vi "LIN_Demo.vi"(11 "Receive":string="LIN_Demo") -> ()   [LabVIEW 2014]
uses:
  TSMaster_API/LIN_Function/Typedef/TSLIN_SendHead.ctl
  <vilib>/Utility/miscctls.llb/LVPointTypeDef.ctl
  TSMaster_API/LIN_Function/Typedef/TLibLIN.ctl
  TSMaster_API/LIN_Function/Typedef/TSLIN_Transmit.ctl
  TSMaster_API/All_Control/Typedef/Hardware Type.ctl
  Utilities/Typedef/Hardware_Subtype.ctl
  TSMaster_API/LIN_Function/Typedef/TSLIN_SetData.ctl
  TSMaster_API/LIN_Function/Typedef/TSLIN_LIN_Set.ctl
  TSMaster_API/All_Control/Typedef/Blf_Log.ctl
  TSMaster_API/LIN_Function/Typedef/TSLIN_LIN Schedule_Table.ctl
  TSMaster_API/LIN_Function/Typedef/TSLIN_Config.ctl
  TSMaster_API/LIN_Function/Typedef/TSLIN_Data.ctl
  TSMaster_API/DataBase/Typedef/FlexRay/TFlexRaySignal.ctl
  TSMaster_API/DataBase/Typedef/LIN/TLINSignal.ctl
  TSMaster_API/DataBase/Typedef/CAN/TCANSignal.ctl
  TSMaster_API/DataBase/Typedef/TDBSignalProperties.ctl
  TSMaster_API/DataBase/Typedef/TDBFrameProperties.ctl
  TSMaster_API/DataBase/Typedef/TDBECUProperties.ctl
  TSMaster_API/DataBase/Typedef/TDBProperties.ctl
  <vilib>/regexp/Match Regular Expression.xnode
  TSMaster_API/DataBase/Typedef/DataBase_array.ctl
  TSMaster_API/DataBase/Typedef/DataBase_array_index.ctl
panel:
  out "DataBase_array":T1
  in  "Diagram shown":bool
  in  "Stop Log":bool
  in  "Start Log":bool
  in  "log":i32(listbox)
  in  "Config":bool
  in  "选项卡控件":enum32{"Setting", "Send&Receie", "LDF_Load"}(tab)
  in  "CH_Mapping":bool
  in  "Set Node":bool
  in  "TS_Mapping":bool
  in  "BLF_Log_PATH":path
  in  "DLL_PATH":path
  in  "Channels used":u16(ring)=1 items=["1 Channel"=1, "2 Channels"=2, "3 Channels"=3, "4 Channels"=4, "5 Channels"=5, "6 Channels"=6, "7 Channels"=7, "8 Channels"=8, "9 Channels"=9, "10 Channels"=10, "11 Channels"=11, "12 Channels"=12, "13 Channels"=13, "14 Channels"=14, "15 Channels"=15, "16 Channels"=16]
  in  "LIN_Data.LIN_Set_Array":T9[](array[typedef]) {"Set_node_funtiontype" items=["MasterNode", "SlaveNode", "MonitorNote"]; "Set"."Hardware Type" items=["BUS_UNKNOWN_TYPE", "TS_TCP_DEVICE", "XL_USB_DEVICE", "TS_USB_DEVICE", "PEAK_USB_DEVICE", "KVASER_USB_DEVICE", "ZLG_USB_DEVICE", "ICS_USB_DEVICE", "TS_TC1005_DEVICE", "CANABLE_USB_DEVICE", "TS_WIRELESS_OBD", "TS_USB_DEVICE_EX", "IXXAT_USB_DEVICE", "TS_ETH_IF_DEVICE", "TS_USB_IF_DEVICE", "BUS_DEV_TYPE_COUNT"]; "Set"."AHwChannel" items=["CHN1", "CHN2", "CHN3", "CHN4", "CHN5", "CHN6", "CHN7", "CHN8", "CHN9", "CHN10", "CHN11", "CHN12", "CHN13", "CHN14", "CHN15", "CHN16", "CHN17", "CHN18", "CHN19", "CHN20", "CHN21", "CHN22", "CHN23", "CHN24", "CHN25", "CHN26", "CHN27", "CHN28", "CHN29", "CHN30", "CHN31", "CHN32"]; "Set"."AAppChannel" items=["CHN1", "CHN2", "CHN3", "CHN4", "CHN5", "CHN6", "CHN7", "CHN8", "CHN9", "CHN10", "CHN11", "CHN12", "CHN13", "CHN14", "CHN15", "CHN16", "CHN17", "CHN18", "CHN19", "CHN20", "CHN21", "CHN22", "CHN23", "CHN24", "CHN25", "CHN26", "CHN27", "CHN28", "CHN29", "CHN30", "CHN31", "CHN32"]; "Set"."AProtocol" items=["Lin_Protocol_13", "Lin_Protocol_20", "Lin_Protocol_21", "Lin_Protocol_J2602"]}
  in  "Export":bool
  in  "Import":bool
  in  "Fold Data":bool
  out "BufferCount":i32
  in  "REC_Channel":i32(ring) items=["CHN1", "CHN2", "CHN3", "CHN4", "CHN5", "CHN6", "CHN7", "CHN8", "CHN9", "CHN10", "CHN11", "CHN12", "CHN13", "CHN14", "CHN15", "CHN16", "CHN17", "CHN18", "CHN19", "CHN20", "CHN21", "CHN22", "CHN23", "CHN24", "CHN25", "CHN26", "CHN27", "CHN28", "CHN29", "CHN30", "CHN31", "CHN32"]
  in  "DIS_REC":bool
  in  "Pause":bool
  in  "Rx/TX":enum16{"Rx", "Tx"}(ring)
  in  "ALINId":u32 format="%.0x"
  in  "ALINDLC":u32 format="%.0x"
  in  "Clear":bool
  in  "LIN_Data_0":i32(listbox)=-1
  in  "LIN_DATA":T13 {"Data7" format="%x"; "Data6" format="%x"; "Data5" format="%x"; "Data4" format="%x"; "Data3" format="%x"; "Data2" format="%x"; "Data1" format="%x"; "Data0" format="%x"}
  in  "Read Message Type":T14(ring)=enum."Receive&send messages"
  out "Receive Status":bool
  out "program loop":i32
  in  "Channel":i32(ring) items=["CHN1", "CHN2", "CHN3", "CHN4", "CHN5", "CHN6", "CHN7", "CHN8", "CHN9", "CHN10", "CHN11", "CHN12", "CHN13", "CHN14", "CHN15", "CHN16", "CHN17", "CHN18", "CHN19", "CHN20", "CHN21", "CHN22", "CHN23", "CHN24", "CHN25", "CHN26", "CHN27", "CHN28", "CHN29", "CHN30", "CHN31", "CHN32"]
  in  "Tag":T15(tab)
  in  "LIN_Schedule_Tab":bool
  in  "Cycle":bool=TRUE
  in  "SendHead&Receive":bool
  out "Successful ?":bool
  in  "ATimeoutMs":i32=200
  in  "Send_Frame":bool
  out "successful ？":bool
  in  "Cycle 2":bool=TRUE
  in  "async&sync":enum16{"async", "sync"}(ring)
  in  "Timeout":u16
  out "Laod LDF Successful?":bool caption="Laod BDC Successful?"
  in  "LDF Tab":enum32{"Message", "Signal"}(tab) caption="Tab Control 2"
  in  "Message Table":string[][](table)=[["Name", ""], ["Data Length", ""], ["Identifier", ""], ["", ""], ["", ""], ["", ""], ["", ""]]
  in  "Signal Table":string[][](table)=[["Name", ""], ["Length", ""], ["Endian", ""], ["DataType", ""], ["FStartBit", ""], ["Factor", ""], ["Offset", ""], ["", ""], ["", ""], ["", ""], ["", ""]]
  in  "Unload":bool
  in  "Load_LDF":bool
  in  "LDF loading channel":i32(ring) items=["CHN1", "CHN2", "CHN3", "CHN4", "CHN5", "CHN6", "CHN7", "CHN8", "CHN9", "CHN10", "CHN11", "CHN12", "CHN13", "CHN14", "CHN15", "CHN16", "CHN17", "CHN18", "CHN19", "CHN20", "CHN21", "CHN22", "CHN23", "CHN24", "CHN25", "CHN26", "CHN27", "CHN28", "CHN29", "CHN30", "CHN31", "CHN32"]
  in  "Tree control":string(tree)
  in  "LDF Path":path
  out "Connect ?":bool
  in  "Disconnect":bool
  in  "Connect":bool
  in  "STOP":bool
  # "LIN_Demo"
  # "Please click the 'Config' button first,Don't click \"Connect\""
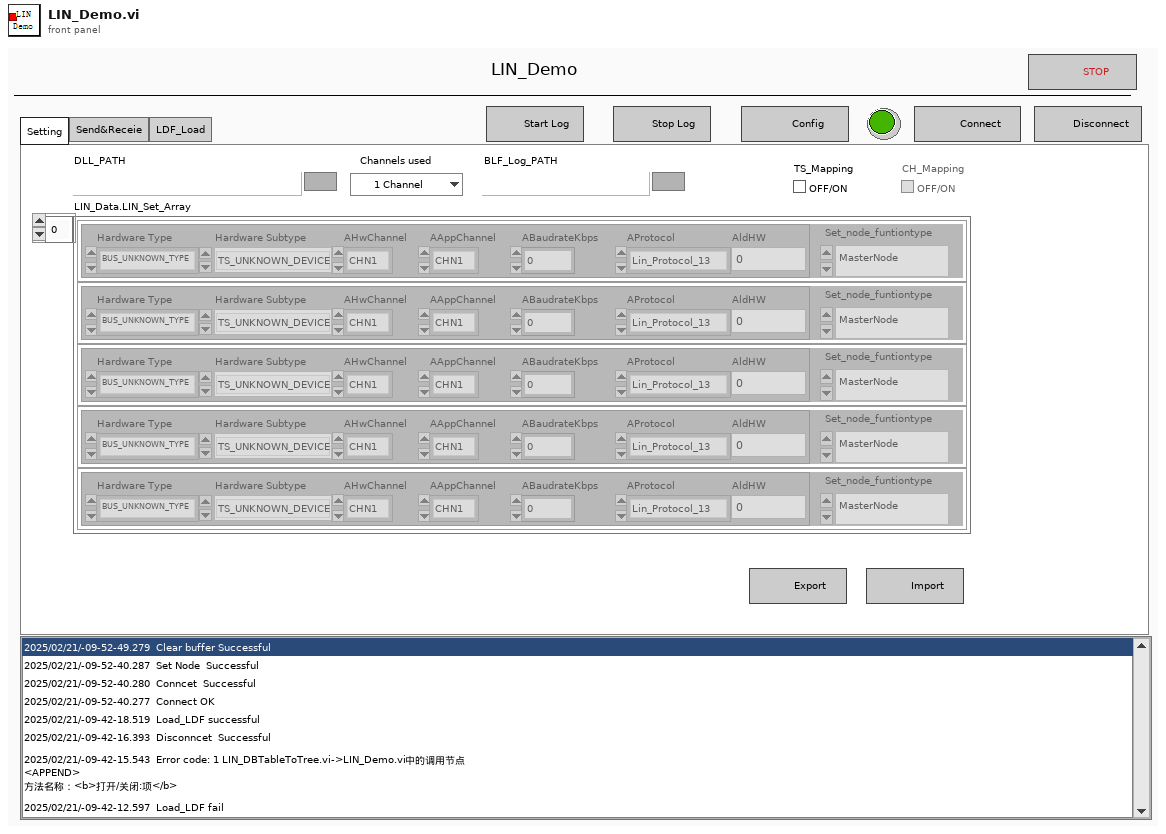
[diagram p1: front panel]
types:
  T1 = typedef "DataBase_array.ctl" = cluster{"db_properties":T2, "ECU_array":cluster{"TDBECUProperties":T3, "TX_Frame_array":cluster{"Frame_Properties":T4, "signal_array":T5[]}[], "RX_Frame_array":cluster{"Frame_Properties":T4, "signal_array":T5[]}[]}[]}[]
  T2 = typedef "TDBProperties.ctl" = cluster{"FDBIndex":i32, "FSignalCount":i32, "FFrameCount":i32, "FECUCount":i32, "FSupportedChannelMask":u64, "FName":cluster{"数值":u64, "数值 2":u64, "数值 3":u64, "数值 4":u64, "数值 5":u64, "数值 6":u64, "数值 7":u64, "数值 8":u64, "数值 9":u64, "数值 10":u64, "数值 11":u64, "数值 12":u64, "数值 13":u64, "数值 14":u64, "数值 15":u64, "数值 16":u64, "数值 17":u64, "数值 18":u64, "数值 19":u64, "数值 20":u64, "数值 21":u64, "数值 22":u64, "数值 23":u64, "数值 24":u64, "数值 25":u64, "数值 26":u64, "数值 27":u64, "数值 28":u64, "数值 29":u64, "数值 30":u64, "数值 31":u64, "数值 32":u64, "数值 33":u64, "数值 34":u64, "数值 35":u64, "数值 36":u64, "数值 37":u64, "数值 38":u64, "数值 39":u64, "数值 40":u64, "数值 41":u64, "数值 42":u64, "数值 43":u64, "数值 44":u64, "数值 45":u64, "数值 46":u64, "数值 47":u64, "数值 48":u64, "数值 49":u64, "数值 50":u64, "数值 51":u64, "数值 52":u64, "数值 53":u64, "数值 54":u64, "数值 55":u64, "数值 56":u64, "数值 57":u64, "数值 58":u64, "数值 59":u64, "数值 60":u64, "数值 61":u64, "数值 62":u64, "数值 63":u64, "数值 64":u64}, "FComment":cluster{"数值":u64, "数值 2":u64, "数值 3":u64, "数值 4":u64, "数值 5":u64, "数值 6":u64, "数值 7":u64, "数值 8":u64, "数值 9":u64, "数值 10":u64, "数值 11":u64, "数值 12":u64, "数值 13":u64, "数值 14":u64, "数值 15":u64, "数值 16":u64, "数值 17":u64, "数值 18":u64, "数值 19":u64, "数值 20":u64, "数值 21":u64, "数值 22":u64, "数值 23":u64, "数值 24":u64, "数值 25":u64, "数值 26":u64, "数值 27":u64, "数值 28":u64, "数值 29":u64, "数值 30":u64, "数值 31":u64, "数值 32":u64, "数值 33":u64, "数值 34":u64, "数值 35":u64, "数值 36":u64, "数值 37":u64, "数值 38":u64, "数值 39":u64, "数值 40":u64, "数值 41":u64, "数值 42":u64, "数值 43":u64, "数值 44":u64, "数值 45":u64, "数值 46":u64, "数值 47":u64, "数值 48":u64, "数值 49":u64, "数值 50":u64, "数值 51":u64, "数值 52":u64, "数值 53":u64, "数值 54":u64, "数值 55":u64, "数值 56":u64, "数值 57":u64, "数值 58":u64, "数值 59":u64, "数值 60":u64, "数值 61":u64, "数值 62":u64, "数值 63":u64, "数值 64":u64}, "FFlags":u32, "FDBId":u32}
  T3 = typedef "TDBECUProperties.ctl" = cluster{"FDBIndex":i32, "FECUIndex":i32, "FTxFrameCount":i32, "FRxFrameCount":i32, "FName":cluster{"数值":u64, "数值 2":u64, "数值 3":u64, "数值 4":u64, "数值 5":u64, "数值 6":u64, "数值 7":u64, "数值 8":u64, "数值 9":u64, "数值 10":u64, "数值 11":u64, "数值 12":u64, "数值 13":u64, "数值 14":u64, "数值 15":u64, "数值 16":u64, "数值 17":u64, "数值 18":u64, "数值 19":u64, "数值 20":u64, "数值 21":u64, "数值 22":u64, "数值 23":u64, "数值 24":u64, "数值 25":u64, "数值 26":u64, "数值 27":u64, "数值 28":u64, "数值 29":u64, "数值 30":u64, "数值 31":u64, "数值 32":u64, "数值 33":u64, "数值 34":u64, "数值 35":u64, "数值 36":u64, "数值 37":u64, "数值 38":u64, "数值 39":u64, "数值 40":u64, "数值 41":u64, "数值 42":u64, "数值 43":u64, "数值 44":u64, "数值 45":u64, "数值 46":u64, "数值 47":u64, "数值 48":u64, "数值 49":u64, "数值 50":u64, "数值 51":u64, "数值 52":u64, "数值 53":u64, "数值 54":u64, "数值 55":u64, "数值 56":u64, "数值 57":u64, "数值 58":u64, "数值 59":u64, "数值 60":u64, "数值 61":u64, "数值 62":u64, "数值 63":u64, "数值 64":u64}, "FComment":cluster{"数值":u64, "数值 2":u64, "数值 3":u64, "数值 4":u64, "数值 5":u64, "数值 6":u64, "数值 7":u64, "数值 8":u64, "数值 9":u64, "数值 10":u64, "数值 11":u64, "数值 12":u64, "数值 13":u64, "数值 14":u64, "数值 15":u64, "数值 16":u64, "数值 17":u64, "数值 18":u64, "数值 19":u64, "数值 20":u64, "数值 21":u64, "数值 22":u64, "数值 23":u64, "数值 24":u64, "数值 25":u64, "数值 26":u64, "数值 27":u64, "数值 28":u64, "数值 29":u64, "数值 30":u64, "数值 31":u64, "数值 32":u64, "数值 33":u64, "数值 34":u64, "数值 35":u64, "数值 36":u64, "数值 37":u64, "数值 38":u64, "数值 39":u64, "数值 40":u64, "数值 41":u64, "数值 42":u64, "数值 43":u64, "数值 44":u64, "数值 45":u64, "数值 46":u64, "数值 47":u64, "数值 48":u64, "数值 49":u64, "数值 50":u64, "数值 51":u64, "数值 52":u64, "数值 53":u64, "数值 54":u64, "数值 55":u64, "数值 56":u64, "数值 57":u64, "数值 58":u64, "数值 59":u64, "数值 60":u64, "数值 61":u64, "数值 62":u64, "数值 63":u64, "数值 64":u64}}
  T4 = typedef "TDBFrameProperties.ctl" = cluster{"FDBIndex":i32, "FECUIndex":i32, "FFrameIndex":i32, "FIsTx":u8, "FReserved1":u8, "FCycleTimeMs":u16, "TSignalType":i32, "FCANIsDataFrame":u8, "FCANIsStdFrame":u8, "FCANIsEdl":u8, "FCANIsBrs":u8, "FCANIdentifier":i32, "FCANDLC":i32, "FCANDataBytes":i32, "FLINIdentifier":i32, "FLINDLC":i32, "FFRChannelMask":u8, "FFRBaseCycle":u8, "FFRCycleRepetition":u8, "FFRIsStartupFrame":u8, "FFRSlotId":u16, "FFRDLC":u16, "FFRCycleMask":u64, "FSignalCount":i32, "FName":cluster{"数值":u64, "数值 2":u64, "数值 3":u64, "数值 4":u64, "数值 5":u64, "数值 6":u64, "数值 7":u64, "数值 8":u64, "数值 9":u64, "数值 10":u64, "数值 11":u64, "数值 12":u64, "数值 13":u64, "数值 14":u64, "数值 15":u64, "数值 16":u64, "数值 17":u64, "数值 18":u64, "数值 19":u64, "数值 20":u64, "数值 21":u64, "数值 22":u64, "数值 23":u64, "数值 24":u64, "数值 25":u64, "数值 26":u64, "数值 27":u64, "数值 28":u64, "数值 29":u64, "数值 30":u64, "数值 31":u64, "数值 32":u64, "数值 33":u64, "数值 34":u64, "数值 35":u64, "数值 36":u64, "数值 37":u64, "数值 38":u64, "数值 39":u64, "数值 40":u64, "数值 41":u64, "数值 42":u64, "数值 43":u64, "数值 44":u64, "数值 45":u64, "数值 46":u64, "数值 47":u64, "数值 48":u64, "数值 49":u64, "数值 50":u64, "数值 51":u64, "数值 52":u64, "数值 53":u64, "数值 54":u64, "数值 55":u64, "数值 56":u64, "数值 57":u64, "数值 58":u64, "数值 59":u64, "数值 60":u64, "数值 61":u64, "数值 62":u64, "数值 63":u64, "数值 64":u64}, "FComment":cluster{"数值":u64, "数值 2":u64, "数值 3":u64, "数值 4":u64, "数值 5":u64, "数值 6":u64, "数值 7":u64, "数值 8":u64, "数值 9":u64, "数值 10":u64, "数值 11":u64, "数值 12":u64, "数值 13":u64, "数值 14":u64, "数值 15":u64, "数值 16":u64, "数值 17":u64, "数值 18":u64, "数值 19":u64, "数值 20":u64, "数值 21":u64, "数值 22":u64, "数值 23":u64, "数值 24":u64, "数值 25":u64, "数值 26":u64, "数值 27":u64, "数值 28":u64, "数值 29":u64, "数值 30":u64, "数值 31":u64, "数值 32":u64, "数值 33":u64, "数值 34":u64, "数值 35":u64, "数值 36":u64, "数值 37":u64, "数值 38":u64, "数值 39":u64, "数值 40":u64, "数值 41":u64, "数值 42":u64, "数值 43":u64, "数值 44":u64, "数值 45":u64, "数值 46":u64, "数值 47":u64, "数值 48":u64, "数值 49":u64, "数值 50":u64, "数值 51":u64, "数值 52":u64, "数值 53":u64, "数值 54":u64, "数值 55":u64, "数值 56":u64, "数值 57":u64, "数值 58":u64, "数值 59":u64, "数值 60":u64, "数值 61":u64, "数值 62":u64, "数值 63":u64, "数值 64":u64}}
  T5 = typedef "TDBSignalProperties.ctl" = cluster{"FDBIndex":i32, "FECUIndex":i32, "FFrameIndex":i32, "FSignalIndex":i32, "FIsTx":u8, "FReserved1":u8, "FReserved2":u8, "FReserved3":u8, "TSignalType":i32, "TCANSignal":T6, "TLINSignal":T7, "TFlexRaySignal":T8, "FParentFrameId":i32, "FInitValue":dbl, "FName":cluster{"数值":u64, "数值 2":u64, "数值 3":u64, "数值 4":u64, "数值 5":u64, "数值 6":u64, "数值 7":u64, "数值 8":u64, "数值 9":u64, "数值 10":u64, "数值 11":u64, "数值 12":u64, "数值 13":u64, "数值 14":u64, "数值 15":u64, "数值 16":u64, "数值 17":u64, "数值 18":u64, "数值 19":u64, "数值 20":u64, "数值 21":u64, "数值 22":u64, "数值 23":u64, "数值 24":u64, "数值 25":u64, "数值 26":u64, "数值 27":u64, "数值 28":u64, "数值 29":u64, "数值 30":u64, "数值 31":u64, "数值 32":u64, "数值 33":u64, "数值 34":u64, "数值 35":u64, "数值 36":u64, "数值 37":u64, "数值 38":u64, "数值 39":u64, "数值 40":u64, "数值 41":u64, "数值 42":u64, "数值 43":u64, "数值 44":u64, "数值 45":u64, "数值 46":u64, "数值 47":u64, "数值 48":u64, "数值 49":u64, "数值 50":u64, "数值 51":u64, "数值 52":u64, "数值 53":u64, "数值 54":u64, "数值 55":u64, "数值 56":u64, "数值 57":u64, "数值 58":u64, "数值 59":u64, "数值 60":u64, "数值 61":u64, "数值 62":u64, "数值 63":u64, "数值 64":u64}, "FComment":cluster{"数值":u64, "数值 2":u64, "数值 3":u64, "数值 4":u64, "数值 5":u64, "数值 6":u64, "数值 7":u64, "数值 8":u64, "数值 9":u64, "数值 10":u64, "数值 11":u64, "数值 12":u64, "数值 13":u64, "数值 14":u64, "数值 15":u64, "数值 16":u64, "数值 17":u64, "数值 18":u64, "数值 19":u64, "数值 20":u64, "数值 21":u64, "数值 22":u64, "数值 23":u64, "数值 24":u64, "数值 25":u64, "数值 26":u64, "数值 27":u64, "数值 28":u64, "数值 29":u64, "数值 30":u64, "数值 31":u64, "数值 32":u64, "数值 33":u64, "数值 34":u64, "数值 35":u64, "数值 36":u64, "数值 37":u64, "数值 38":u64, "数值 39":u64, "数值 40":u64, "数值 41":u64, "数值 42":u64, "数值 43":u64, "数值 44":u64, "数值 45":u64, "数值 46":u64, "数值 47":u64, "数值 48":u64, "数值 49":u64, "数值 50":u64, "数值 51":u64, "数值 52":u64, "数值 53":u64, "数值 54":u64, "数值 55":u64, "数值 56":u64, "数值 57":u64, "数值 58":u64, "数值 59":u64, "数值 60":u64, "数值 61":u64, "数值 62":u64, "数值 63":u64, "数值 64":u64}}
  T6 = typedef "TCANSignal.ctl" = cluster{"FCANSgnType":u8, "FIsIntel":u8, "FStartBit":i32, "FLength":i32, "FFactor":dbl, "FOffset":dbl}
  T7 = typedef "TLINSignal.ctl" = cluster{"FLINSgnType":u8, "FIsIntel":u8, "FStartBit":i32, "FLength":i32, "FFactor":dbl, "FOffset":dbl}
  T8 = typedef "TFlexRaySignal.ctl" = cluster{"FFRSgnType":u8, "FCompuMethod":u8, "FReserved":u8, "FIsIntel":u8, "FStartBit":i32, "FUpdateBit":i32, "FLength":i32, "FFactor":dbl, "FOffset":dbl, "FActualStartBit":i32, "FActualUpdateBit":i32}
  T9 = typedef "TSLIN_LIN_Set.ctl" = cluster{"Set":T10, "Set_node_funtiontype":i32}
  T10 = typedef "TSLIN_SetData.ctl" = cluster{"Hardware Type":T11, "Hardware Subtype":T12, "AHwChannel":i32, "AAppChannel":i32, "ABaudrateKbps":sgl, "AProtocol":i32, "AldHW":i32}
  T11 = typedef "Hardware Type.ctl" = i32
  T12 = typedef "Hardware_Subtype.ctl" = enum16{"TS_UNKNOWN_DEVICE", "TSCAN_PRO", "TSCAN_Lite1", "TC1001", "TL1001", "TC1011", "TM5011", "TC1002", "TC1014", "TSCANFD2517", "TC1026", "TC1016", "TC1012", "TC1013", "TLog1002", "TC1034", "TC1018", "GW2116", "TC2115", "MP1013", "TC1113", "TC1114", "TP1013", "TC1017", "TP1018", "TF10XX", "TL1004_FD_4_LIN_2", "TE1051", "TP1051", "TP1034", "TTS9015", "TP1026", "TTS1026", "TTS1034", "TTS1018", "TL1011", "TTS1015_LiAuto", "TTS1013_LiAuto", "TTS1016Pro", "TC1054Pro", "TC1054", "TLog1038", "TO1013", "TC1034Pro", "TC1018Pro", "TC1038Pro", "TS_DEV_END"}
  T13 = cluster{"Data0":u8, "Data1":u8, "Data2":u8, "Data3":u8, "Data4":u8, "Data5":u8, "Data6":u8, "Data7":u8}
  T14 = enum16{"Only read received messages", "Receive&send messages"}
  T15 = enum32{"Schedule Table", "SendHead", "SendFrame"}
  T16 = typedef "TLibLIN.ctl" = cluster{"Ch":u8, "Code":u8, "Properties":u8, "FDLC":u8, "ID":u8, "Checksum":u8, "FStaus":u8, "FTimeUS":u64, "FDatas":cluster{"value0":u8, "value 1":u8, "value 2":u8, "value 3":u8, "value 4":u8, "value 5":u8, "value 6":u8, "value 7":u8}}
  T17 = enum8{"Enabled", "Disabled", "Disabled and Grayed Out"}
  T18 = typedef "TSLIN_Data.ctl" = cluster{"Communication message":cluster{"Sender":string, "receiver":string, "message":string, "data":variant}, "LIN_Data":T19, "LIN Data array":T16[], "error in":errorcluster, "REC_Channel":i32, "AsynCall?":bool, "DataBase_array":T24}
  T19 = typedef "TSLIN_Config.ctl" = cluster{"DLL_PATH":path, "Channels used":u16, "Funtiontype":i32, "Rx/TX":enum16{"Rx", "Tx"}, "Read message type":enum16{"Only read received messages", "Receive&send messages"}, "async&sync":enum16{"async", "sync"}, "sync_sendTimeout":u16, "LIN_SendHead":T20, "LIN_Set":T10, "LIN_DATA":cluster{"Data0":u8, "Data1":u8, "Data2":u8, "Data3":u8, "Data4":u8, "Data5":u8, "Data6":u8, "Data7":u8}, "LIN_Set_Array":T9[], "LDF":cluster{"LDF Path":path, "LDF loading channel":i32}, "Blf_Log":T21, "LIN Scheduling Table Array":T22[], "REC_Channel":i32}
  T20 = typedef "TSLIN_SendHead.ctl" = cluster{"ALINIdxchn":u8, "ALINId":u32, "ALINDLC":u32}
  T21 = typedef "Blf_Log.ctl" = cluster{"Blf_Log_PATH":path}
  T22 = typedef "TSLIN_LIN Schedule_Table.ctl" = cluster{"LIN_Transmit":T23, "Delay(ms)":i32}
  T23 = typedef "TSLIN_Transmit.ctl" = cluster{"Channel":i32, "Rx/TX":enum16{"Rx", "Tx"}, "Set_node_funtiontype":i32, "DLC":u32, "ID":u32, "FDatas":cluster{"value0":u8, "value 1":u8, "value 2":u8, "value 3":u8, "value 4":u8, "value 5":u8, "value 6":u8, "value 7":u8}}
  T24 = typedef "DataBase_array_index.ctl" = refnum<vi>
  T25 = typedef "LVPointTypeDef.ctl" = cluster{"Horizontal":i16, "Vertical":i16}
  T26 = cluster{"Sender":string, "receiver":string, "message":string, "data":variant, "LIN Data array":T16[]}
  T27 = cluster{"Sender":string, "receiver":string, "message":string, "data":variant}
  T28 = cluster{"Frame_Properties":T4, "signal_array":T5[]}
  T29 = enum32{"invalid app kind", "Development System", "Run Time System", "Student Edition", "Embedded LabVIEW", "Evaluation", "Custom"}
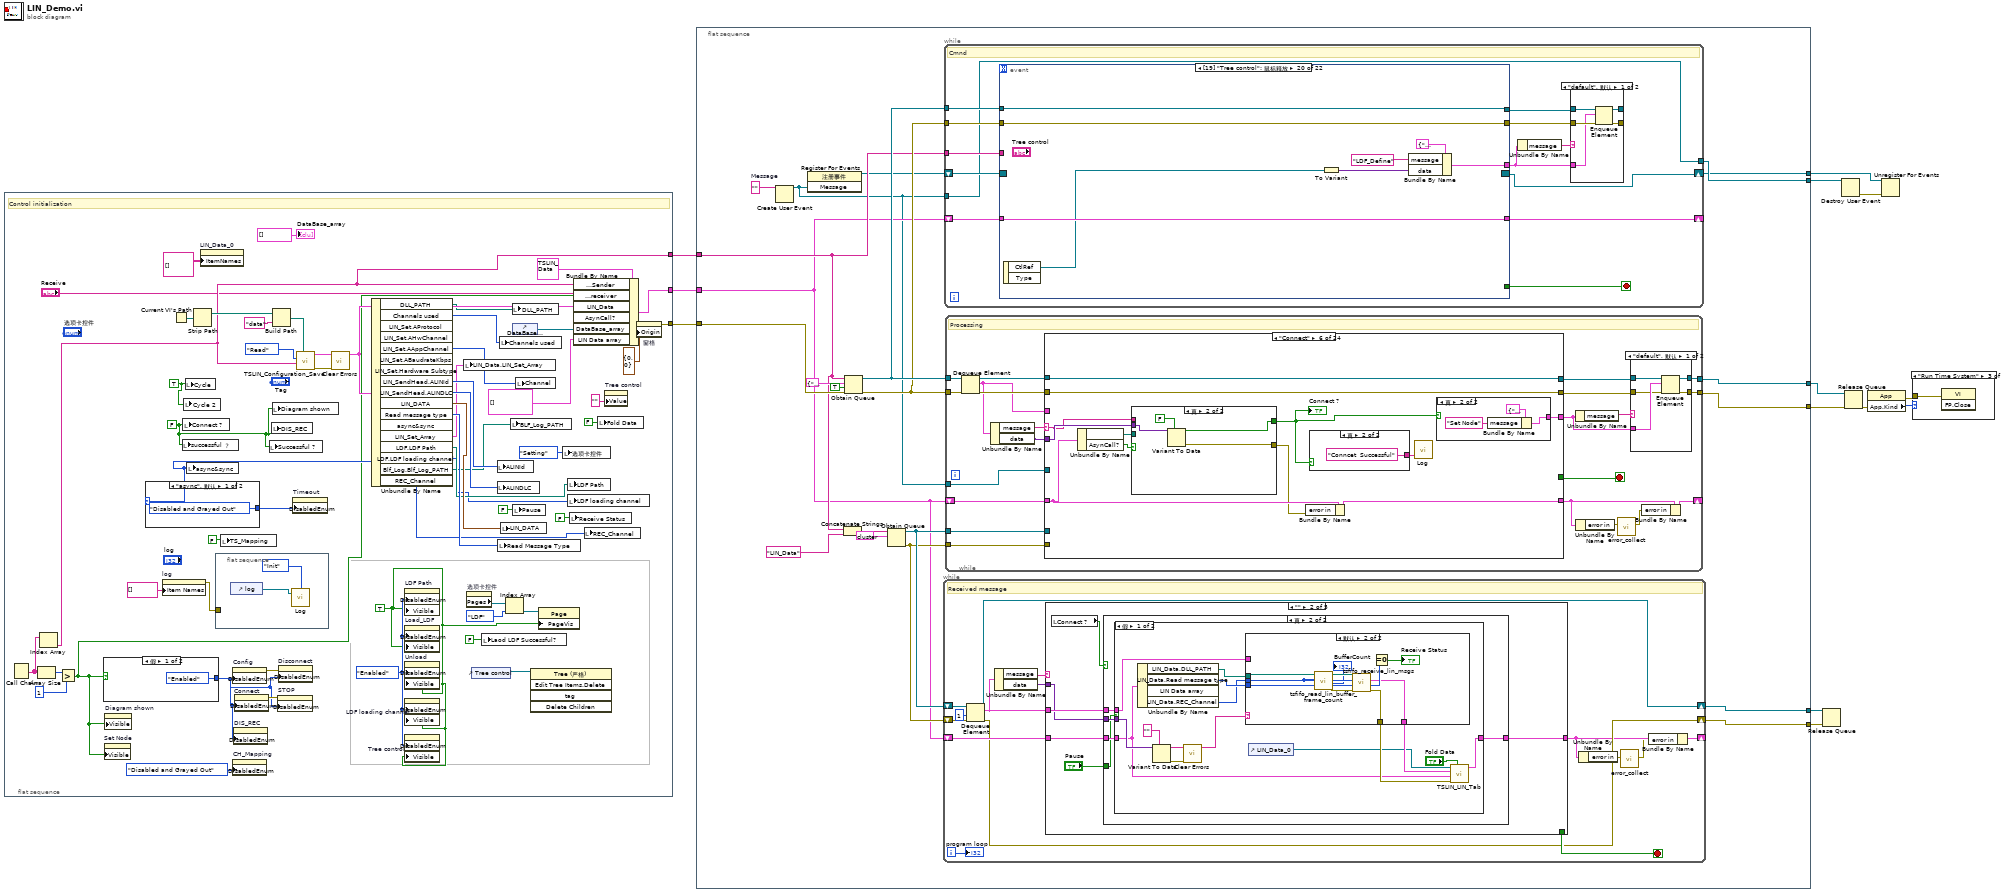
[diagram p0: block diagram]
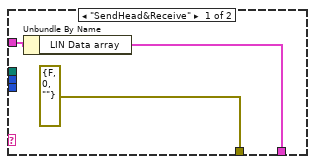
[diagram p4: hidden frame]
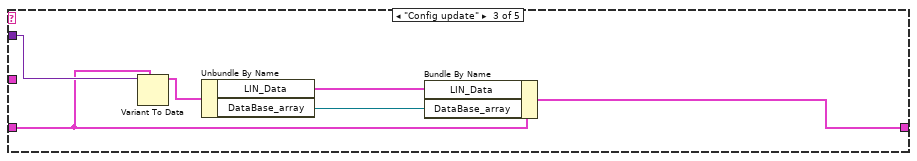
[diagram p6: hidden frame]
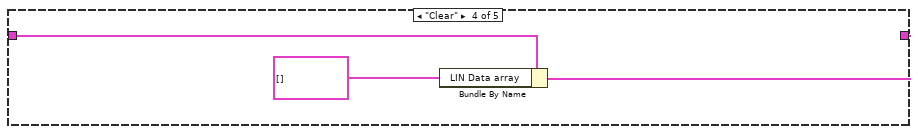
[diagram p7: hidden frame]
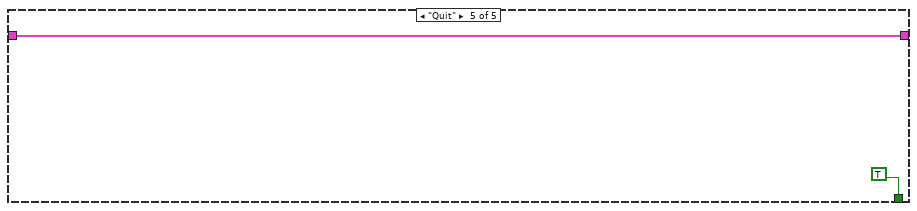
[diagram p8: hidden frame]
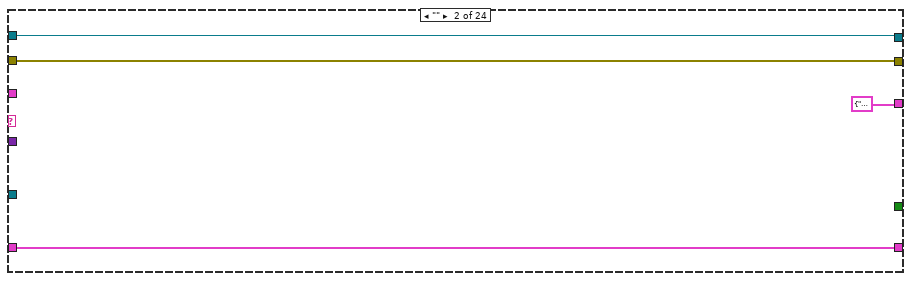
[diagram p11: hidden frame]
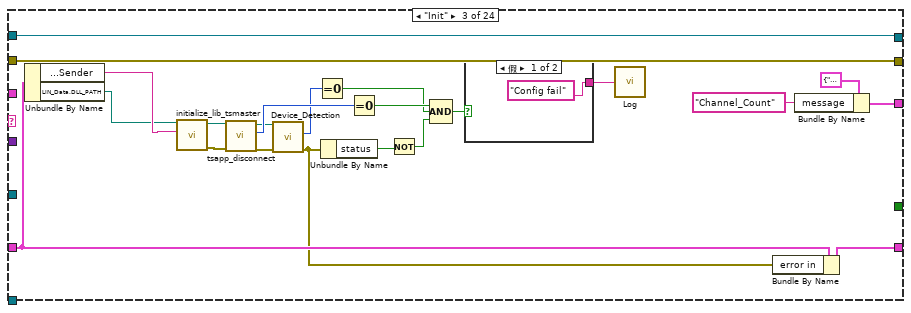
[diagram p12: hidden frame]
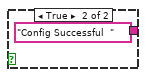
[diagram p13: hidden frame]
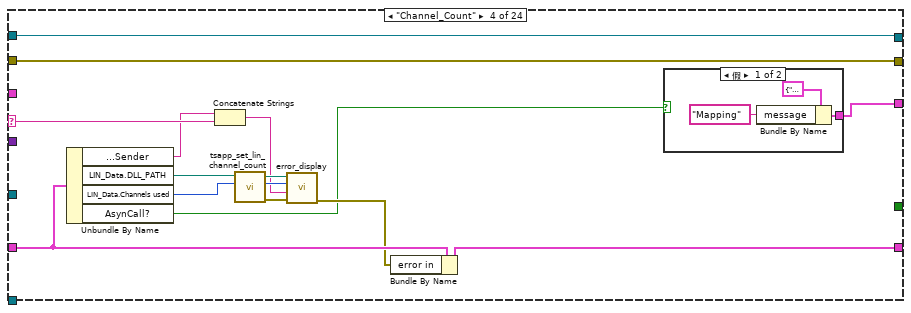
[diagram p14: hidden frame]
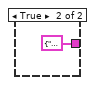
[diagram p15: hidden frame]
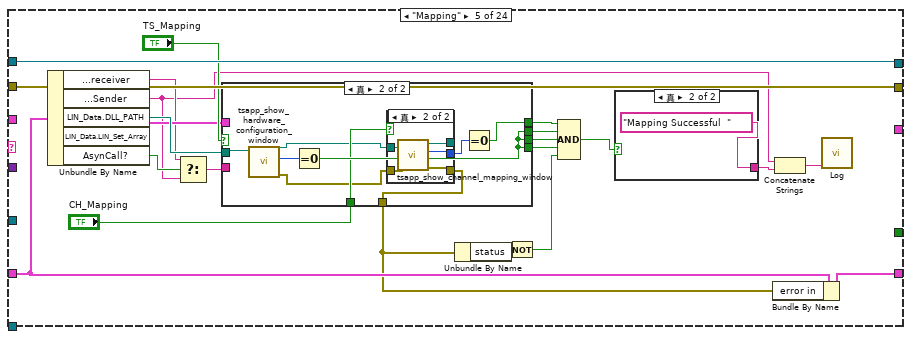
[diagram p16: hidden frame]
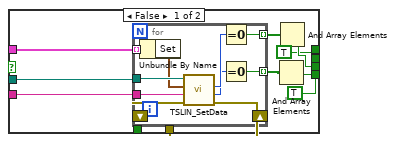
[diagram p17: hidden frame]
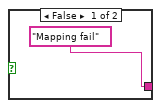
[diagram p19: hidden frame]
diagram:
  n1 = flat-sequence {
    tunnel: [w66] -> w13
    tunnel: [w25] -> w12
    tunnel: [w62] -> w11
    frame #0 {
      w33 = TRUE
      w42 = T17."Enabled" ("禁用")
      w59 = TRUE ("Cycle")
      w27 = FALSE ("Connect ?")
      # "Control initialization"
      n2 = Call Chain() -> (call chain=w26:string[])
      n3 = Array Size(array=w26) -> (size(s)=w29:i32)
      n4 = Index Array(array=w26) -> (element=w25:string)  [unwired: 1 in]
      n5 = Greater?(x=w29, y=1) -> (0:w22:bool)
      n6 = case shown="假" w22 {
        tunnel: [T17."Enabled" ("禁用") T17."Disabled and Grayed Out" ("禁用")] -> w23
        frame False {
        }
        frame True {
        }
      }
      n7 = property on="Set Node" class="Bool"("Visible"=w22) -> ()  [unwired: 2 in, 2 out]
      n8 = property on="Diagram shown" class="Bool (严格)"("Visible"=w22) -> ()  [unwired: 2 in, 2 out]
      n9 = property on="log" class="LstBox (严格)"("Item Names"=string[] [] ("项名")) -> (error out=w40:errorcluster)  [unwired: 2 in, 1 out]
      n10 = Current VI's Path() -> (path=w55:path)
      n11 = local write "successful ？"(w27) -> ()
      n12 = local write "Connect ?"(w27) -> ()
      n13 = local write "Cycle 2"(w59) -> ()
      n14 = local write "Cycle"(w59) -> ()
      n15 = Strip Path(path=w55) -> (stripped path=w53:path)  [unwired: 1 out]
      n16 = property on="LIN_Data_0" class="MCListbox (严格)"("ItemNames"=string[][] [] ("项名")) -> ()  [unwired: 2 in, 2 out]
      n17 = flat-sequence {
        tunnel: w40 -> [_]
        frame #0 {
          n18 = control-ref of="log"() -> (w73:refnum<vi>)
          n19 = call "Log.vi"("Method"=enum16{"Init", "Log"}."Init", "ListBox in"=w73) -> ()  [unwired: 2 in]
        }
      }
      n20 = local write "TS_Mapping"(FALSE ("TS_Mapping")) -> ()
      n21 = property on="Config" class="Bool"("DisabledEnum"=w23) -> (error out=w31:errorcluster)  [unwired: 2 in, 1 out]
      n22 = property on="CH_Mapping" class="Bool (严格)"("DisabledEnum"=T17."Disabled and Grayed Out" ("禁用")) -> ()  [unwired: 2 in, 2 out]
      n23 = property on="DIS_REC" class="Bool (严格)"("DisabledEnum"=w23) -> ()  [unwired: 2 in, 2 out]
      n24 = property on="Connect" class="Bool"("DisabledEnum"=w23) -> (error out=w30:errorcluster)  [unwired: 2 in, 1 out]
      n25 = local write "Successful ?"(w27) -> ()
      n26 = local write "DIS_REC"(w27) -> ()
      n27 = local write "Diagram shown"(w27) -> ()
      n28 = Build Path(base path=w53, name or relative path="data") -> (appended path=w52:path)
      n29 = property on="STOP" class="Bool"(error in=w30, "DisabledEnum"=w23) -> ()  [unwired: 1 in, 2 out]
      n30 = property on="Disconnect" class="Bool"(error in=w31, "DisabledEnum"=w23) -> ()  [unwired: 1 in, 2 out]
      n31 = call "TSLIN_Configuration_Save.vi"("path"=w52, "Config Name"=w25, "Read/Write"=enum16{"Read", "Write"}."Read") -> ("error in (no error) 2"=w48:errorcluster, "LIN_Data out"=w67:T19)  [unwired: 6 in, 1 out]
      n32 = call <vilib>:"Clear Errors.vi"("error in (no error)"=w48) -> ()  [unwired: 5 in, 2 out]
      n33 = Unbundle By Name(w67) -> ("DLL_PATH"=w49:path, "Channels used"=w50:u16, "LIN_Set.AAppChannel"=w68:i32, "LIN_SendHead.ALINId"=w64:u32, "LIN_SendHead.ALINDLC"=w63:u32, "LIN_DATA"=w61:T13, "Read message type"=w57:T14, "async&sync"=w56:enum16{"async", "sync"}, "LIN_Set_Array"=w47:T9[], "LDF.LDF Path"=w45:path, "LDF.LDF loading channel"=w44:i32, "Blf_Log.Blf_Log_PATH"=w36:path, "REC_Channel"=w32:i32)  [unwired: 4 out]
      n34 = case shown="\"async\", 默认" w56 {
        tunnel: [T17."Disabled and Grayed Out" ("禁用") T17."Enabled" ("禁用")] -> w58
        frame "async", Default {
        }
        frame "sync" {
        }
      }
      n35 = local write "async&sync"(w56) -> ()
      n36 = property on="Timeout" class="DigNum (严格)"("DisabledEnum"=w58) -> ()  [unwired: 2 in, 2 out]
      n37 = property on="LDF Path" class="Path"("DisabledEnum"=w42, "Visible"=w33) -> ()  [unwired: 2 in, 2 out]
      n38 = property on="Load_LDF" class="Bool"("DisabledEnum"=w42, "Visible"=w33) -> ()  [unwired: 2 in, 2 out]
      n39 = property on="Unload" class="Bool"("DisabledEnum"=w42, "Visible"=w33) -> ()  [unwired: 2 in, 2 out]
      n40 = property on="LDF loading channel" class="Ring (严格)"("DisabledEnum"=w42, "Visible"=w33) -> ()  [unwired: 2 in, 2 out]
      n41 = property on="Tree control" class="Tree (严格)"("DisabledEnum"=w42, "Visible"=w33) -> ()  [unwired: 2 in, 2 out]
      n42 = local write "LIN_Data.LIN_Set_Array"(w47) -> ()
      n43 = property on="选项卡控件" class="TabCtl (严格)"() -> ("Pages"=w39:refnum<vi>[])  [unwired: 2 in, 2 out]
      n44 = control-ref of="Tree control"() -> (w15:refnum<vi>)
      n45 = local write "Laod LDF Successful?"(FALSE ("Laod LDF Successful?")) -> ()
      n46 = local write "ALINId"(w64) -> ()
      n47 = local write "ALINDLC"(w63) -> ()
      n48 = local write "Read Message Type"(w57) -> ()
      n49 = local write "Channels used"(w50) -> ()
      n50 = local write "LIN_DATA"(w61) -> ()
      n51 = Index Array(array=w39, index=enum32{"Setting", "Send&Receie", "LDF"}."LDF" ("选项卡控件")) -> (element=w37:refnum<vi>)
      n52 = local write "BLF_Log_PATH"(w36) -> ()
      n53 = local write "DLL_PATH"(w49) -> ()
      n54 = control-ref of="DataBase_array"() -> (w16:refnum<vi>)
      n55 = local write "Pause"(FALSE ("Pause")) -> ()
      n56 = local write "Channel"(w68) -> ()
      n57 = invoke class="Tree (严格)" method="Edit Tree Items.Delete"(reference=w15) -> ()  [unwired: 4 in, 5 out]
      n58 = property class="Page"(reference=w37, "PageVis"=w33) -> ()  [unwired: 1 in, 2 out]
      n59 = local write "选项卡控件"(enum32{"Setting", "Send&Receie", "LDF_Load"}."Setting" ("选项卡控件")) -> ()
      n60 = local write "LDF Path"(w45) -> ()
      n61 = local write "LDF loading channel"(w44) -> ()
      n62 = local write "Receive Status"(FALSE ("Receive Status")) -> ()
      n63 = Bundle By Name(cluster=T18 {"Communication message"={"Sender"="", "receiver"="", "message"="", "data"=variant}, "LIN_Data"={"DLL_PATH"=path "", "Channels used"=0, "Funtiontype"=0, "Rx/TX"=enum."Rx", "Read message type"=enum."Only read received messages", "async&sync"=enum."async", "sync_sendTimeout"=0, "LIN_SendHead"={"ALINIdxchn"=0, "ALINId"=0, "ALINDLC"=0}, "LIN_Set"={"Hardware Type"=0, "Hardware Subtype"=enum."TS_UNKNOWN_DEVICE", "AHwChannel"=0, "AAppChannel"=0, "ABaudrateKbps"=0.0, "AProtocol"=0, "AldHW"=0}, "LIN_DATA"={"Data0"=0, "Data1"=0, "Data2"=0, "Data3"=0, "Data4"=0, "Data5"=0, "Data6"=0, "Data7"=0}, "LIN_Set_Array"=[], "LDF"={"LDF Path"=path "", "LDF loading channel"=0}, "Blf_Log"={"Blf_Log_PATH"=path ""}, "LIN Scheduling Table Array"=[], "REC_Channel"=0}, "LIN Data array"=[], "error in"={"status"=FALSE, "code"=0, "source"=""}, "REC_Channel"=0, "AsynCall?"=FALSE, "DataBase_array"=refnum} ("Data"), "Communication message.Sender"=w25, "Communication message.receiver"="Receive", "LIN_Data"=w67, "AsynCall?"=w22, "DataBase_array"=w16, "LIN Data array"=T16[] []) -> (w62:T18)
      n64 = local write "REC_Channel"(w32) -> ()
      n65 = local write "Fold Data"(FALSE ("Fold Data")) -> ()
      n66 = property on="Tree control" class="Tree (严格)"("Value"="" ("Tree control")) -> ()  [unwired: 2 in, 2 out]
      n67 = property on="窗格" class="Pane"("Origin"=T25 {"Horizontal"=0, "Vertical"=0} ("原点")) -> (error out=w66:errorcluster)  [unwired: 2 in, 1 out]
      "DataBase_array" <- T1 [] ("DataBase_array")
    }
  }
  n68 = flat-sequence {
    tunnel: w13 -> [w95]
    tunnel: w12 -> [w89]
    tunnel: w11 -> [w84]
    tunnel: [w81] -> w9
    tunnel: [w80] -> w8
    tunnel: [w79] -> w5
    tunnel: [w78] -> w4
    tunnel: [w77] -> w2
    tunnel: [w76] -> w1
    frame #0 {
      w96 = ""  # Message
      n69 = Create User Event(user event datatype=w96) -> (user event=w82:refnum<user-event>)  [unwired: 1 in, 1 out]
      n70 = register-events(w82) -> (reference out=w83:refnum<event-registration>)  [unwired: 2 in, 1 out]
      n71 = Concatenate Strings(w89, "LIN_Data" ("字符串")) -> (w88:string)
      n72 = Obtain Queue(name (unnamed)=w89, element data type=T27 {"Sender"="", "receiver"="", "message"="", "data"=variant} ("Communication message"), create if not found? (T)=TRUE ("如未找到则创建？(T)"), error in (no error)=w95) -> (queue out=w94:refnum<queue>, error out=w93:errorcluster)  [unwired: 1 in, 1 out]
      n73 = Obtain Queue(name (unnamed)=w88, element data type=T26 {"Sender"="", "receiver"="", "message"="", "data"=variant, "LIN Data array"=[]} ("Communication message")) -> (queue out=w86:refnum<queue>, error out=w85:errorcluster)  [unwired: 3 in, 1 out]
      n74 = while {
        shift-right: [w103] -> w79
        shift-left: w86 -> [w111]
        shift-right: [w102] -> w78
        shift-left: w85 -> [w109]
        shift-right: [w98] -> _
        shift-left: w84 -> [w105]
        i -> [w101]
        stop <- w106 stop-if-true
        # "Received message"
        n75 = Dequeue Element(queue=w111, timeout in ms (-1)=1 ("超时毫秒(-1)"), error in (no error)=w109) -> (queue out=w103:refnum<queue>, element=w104:T26, error out=w102:errorcluster)  [unwired: 1 out]
        n76 = Unbundle By Name(w104) -> ("message"=w108:string, "data"=w107:variant)
        n77 = case shown="\"\"" w108 {
          tunnel: w107 -> [_ w114 w158 _ _]
          tunnel: [_ _ _ _ TRUE] -> w106
          tunnel: w105 -> [w112 w117 w157 w160 w162]
          tunnel: [w112 w116 w156 w159 w162] -> w99
          tunnel: w104 -> [_ w115 _ _ _]
          frame "假", Default {
          }
          frame "" {
            n78 = local read "Connect ?"() -> (w118:bool)
            n79 = case shown="真" w118 {
              tunnel: w117 -> [w119 w121]
              tunnel: [w119 w124] -> w116
              tunnel: w115 -> [_ w123]
              tunnel: w114 -> [_ w122]
              tunnel: "Pause" -> [_ w120]
              frame False {
              }
              frame True {
                n80 = case shown="假" w120 {
                  tunnel: [w136 w152] -> w124
                  tunnel: w123 -> [w135 _]
                  tunnel: w122 -> [w134 _]
                  tunnel: w121 -> [w128 w152]
                  frame False {
                    n81 = Unbundle By Name(w128) -> ("LIN_Data.DLL_PATH"=w138:path, "LIN_Data.Read message type"=w137:T14, "LIN_Data.REC_Channel"=w126:i32)  [unwired: 1 out]
                    n82 = Variant To Data(type="", Variant=w134) -> (data=w132:string, error out=w131:errorcluster)  [unwired: 1 in]
                    n83 = call <vilib>:"Clear Errors.vi"("error in (no error)"=w131) -> ()  [unwired: 5 in, 2 out]
                    n84 = case shown="默认" w132 {
                      tunnel: w138 -> [_ w146]
                      tunnel: w126 -> [_ w144]
                      tunnel: w137 -> [_ w151]
                      tunnel: [w140 w147] -> w130
                      tunnel: w135 -> [w141 _]
                      tunnel: [errorcluster {"status"=FALSE, "code"=0, "source"=""} ("error out") w149] -> w129
                      frame "SendHead&Receive" {
                        n85 = Unbundle By Name(w141) -> ("LIN Data array"=w140:T16[])
                      }
                      frame Default {
                        n86 = call "tsfifo_read_lin_buffer_frame_count.vi"("AAppChannel"=w144, "路径输入"=w146) -> ("错误输出"=w143:errorcluster, "ACount"=→"BufferCount":i32, "路径输出"=w145:path)  [unwired: 6 in, 1 out]
                        n87 = call "tsfifo_receive_lin_msgs.vi"("错误输入（无错误）"=w143, "Read message type"=w151, "AIdxChn"=w144, "路径输入"=w145) -> ("错误输出"=w149:errorcluster, "return"=w150:i32, "ALINBuffer"=w147:T16[])  [unwired: 4 in, 1 out]
                        n88 = Equal To 0?(x=w150) -> (x = 0?=→"Receive Status":bool)
                      }
                    }
                    n89 = control-ref of="LIN_Data_0"() -> (w127:refnum<vi>)
                    n90 = call "TSLIN_LIN_Tab.vi"("Fold Data"="Fold Data", "error in (no error)"=w129, "Data in"=w128, "ALINBuffer"=w130, "MulticolumnListbox in"=w127) -> ("Data out"=w136:T18)  [unwired: 6 in]
                  }
                  frame True {
                  }
                }
              }
            }
          }
          frame "Config update" {
            n91 = Variant To Data(type=w157, Variant=w158) -> (data=w155:T18)  [unwired: 1 in, 1 out]
            n92 = Unbundle By Name(w155) -> ("LIN_Data"=w154:T19, "DataBase_array"=w153:T24)
            n93 = Bundle By Name(cluster=w157, "LIN_Data"=w154, "DataBase_array"=w153) -> (w156:T18)
          }
          frame "Clear" {
            n94 = Bundle By Name(cluster=w160, "LIN Data array"=T16[] []) -> (w159:T18)
          }
          frame "Quit" {
          }
        }
        n95 = Unbundle By Name(w99) -> ("error in"=w100:errorcluster)
        n96 = call "error_collect.vi"("error in (no error)"=w100) -> ("error IO"=w97:errorcluster)  [unwired: 10 in]
        n97 = Bundle By Name(cluster=w99, "error in"=w97) -> (w98:T18)
        "program loop" <- w101
      }
      n98 = while {
        tunnel: w94 -> [w1045]
        tunnel: w93 -> [w1043]
        tunnel: w89 -> [w1039]
        shift-right: [w1036] -> _
        shift-left: w84 -> [w1037]
        shift-right: [w1035] -> w76
        shift-left: w83 -> [w1038]
        tunnel: w82 -> [w1034]
        tunnel: [w1034] -> w77
        stop <- w1046 stop-if-true
        # "Cmnd"
        n99 = event shown="[19] \"Tree control\": 鼠标释放" {
          selector: w1038 -> [_ _ _ _ _ _ _ _ _ _ _ _ _ _ _ _ _ _ _ _ _ _]
          dyn-events: [_ _ _ _ _ _ _ _ _ _ _ _ _ _ _ _ _ _ _ _ _ _] -> w1035
          timeout: _ -> [_ _ _ _ _ _ _ _ _ _ _ _ _ _ _ _ _ _ _ _ _ _]
          tunnel: [_ _ _ _ _ _ _ _ _ _ _ _ _ _ _ _ _ _ w1196 _ w1214 TRUE ("放弃？")] -> w1046
          tunnel: w1045 -> [w1056 w1063 w1069 w1074 w1080 w1084 w1092 w1104 w1113 w1121 w1125 w1151 w1161 w1167 w1173 w1179 w1185 w1192 w1199 w1207 w1213 w1218]
          tunnel: [w1056 w1063 w1069 w1074 w1080 w1084 w1092 w1104 w1113 w1121 w1125 w1151 w1161 w1167 w1173 w1179 w1185 w1192 w1199 w1207 w1213 w1218] -> w1044
          tunnel: [_ w1061 w1064 _ T27 {"Sender"="", "receiver"="", "message"="Connect", "data"=variant} ("Communication message") T27 {"Sender"="", "receiver"="", "message"="Disconnect", "data"=variant} ("Communication message") w1086 w1100 w1108 w1116 T27 {"Sender"="", "receiver"="", "message"="Clear", "data"=variant} ("Communication message") w1144 w1156 w1163 w1168 w1174 w1180 w1187 T27 {"Sender"="", "receiver"="", "message"="eee", "data"=variant} ("Communication message") w1201 w1209 T27 {"Sender"="", "receiver"="", "message"="Quit", "data"=variant} ("Communication message")] -> w1041
          tunnel: [w1055 w1057 w1068 w1073 w1079 w1083 w1091 w1103 w1112 w1120 w1124 w1140 w1160 w1166 w1172 w1178 w1184 w1191 w1194 w1206 w1211 w1216] -> w1042
          tunnel: w1043 -> [w1055 w1057 w1068 w1073 w1079 w1083 w1091 w1103 w1112 w1120 w1124 w1140 w1160 w1166 w1172 w1178 w1184 w1191 w1194 w1206 w1211 w1216]
          tunnel: w1039 -> [_ _ _ _ _ _ _ _ _ _ _ _ _ _ _ _ _ _ _ _ _ _]
          tunnel: w1037 -> [w1054 w1058 w1067 w1072 w1078 w1082 w1090 w1102 w1111 w1119 w1123 w1150 w1159 w1165 w1171 w1177 w1183 w1190 w1195 w1205 w1212 w1217]
          tunnel: [w1054 w1058 w1067 w1072 w1078 w1082 w1090 w1102 w1111 w1119 w1123 w1143 w1159 w1165 w1171 w1177 w1183 w1190 w1195 w1205 w1212 w1217] -> w1036
          event Timeout {
            n100 = event-data() -> ()  [unwired: 1 in, 3 out]
          }
          event "Config": Value Change {
            n101 = event-data() -> ()  [unwired: 1 in, 1 out]
            n102 = To Variant(anything=w1058) -> (Variant=w1059:variant)
            n103 = Bundle By Name(cluster=T27 {"Sender"="", "receiver"="", "message"="", "data"=variant} ("Communication message"), "message"="Init", "data"=w1059) -> (w1061:T27)
          }
          event "Set Node": Value Change {
            n104 = event-data() -> ()  [unwired: 1 in, 1 out]
            n105 = Bundle By Name(cluster=T27 {"Sender"="", "receiver"="", "message"="", "data"=variant} ("Communication message"), "message"="Set Node") -> (w1064:T27)
          }
          event "TS_Mapping": Value Change {
            n106 = event-data() -> ("NewVal"=w1070:bool)  [unwired: 1 in]
            n107 = case shown="假" w1070 {
              tunnel: [T17."Disabled and Grayed Out" ("禁用") T17."Enabled" ("禁用")] -> w1071
              frame False {
              }
              frame True {
              }
            }
            n108 = property on="CH_Mapping" class="Bool (严格)"("DisabledEnum"=w1071) -> ()  [unwired: 2 in, 2 out]
          }
          event "Connect": Value Change {
            n109 = event-data() -> ()  [unwired: 1 in, 1 out]
          }
          event "Disconnect": Value Change {
            n110 = event-data() -> ()  [unwired: 1 in, 1 out]
          }
          event "DIS_REC": Value Change {
            n111 = event-data() -> ("NewVal"=w1085:bool)  [unwired: 1 in, 5 out]
            n112 = To Variant(anything=w1085) -> (Variant=w1087:variant)
            n113 = Bundle By Name(cluster=T27 {"Sender"="", "receiver"="", "message"="", "data"=variant} ("Communication message"), "message"="DIS_REC", "data"=w1087) -> (w1086:T27)
          }
          event "SendHead&Receive": Value Change {
            n114 = event-data() -> ()  [unwired: 1 in, 1 out]
            n115 = property on="Rx/TX" class="Enum (严格)"("Val(Sgnl)"=enum16{"Rx", "Tx"}."Rx" ("值(信号)")) -> ()  [unwired: 2 in, 2 out]
            n116 = Select(t=T17."Disabled and Grayed Out" ("禁用"), s="Cycle", f=T17."Enabled" ("禁用")) -> (s? t:f=w1096:T17)
            n117 = To Variant(anything="Cycle") -> (Variant=w1098:variant)
            n118 = property on="REC_Channel" class="Ring (严格)"("DisabledEnum"=w1096) -> ()  [unwired: 2 in, 2 out]
            n119 = Bundle By Name(cluster=T27 {"Sender"="", "receiver"="", "message"="SendHead&Receive", "data"=variant} ("Communication message"), "message"="SendHead&Receive", "data"=w1098) -> (w1100:T27)
          }
          event "Send_Frame": Value Change {
            # "点击后，若发送成功显示闪烁\nAfter clicking, if the sending is successful, it will flash"
            n120 = event-data() -> ()  [unwired: 1 in, 1 out]
            n121 = property on="Rx/TX" class="Enum (严格)"("Val(Sgnl)"=enum16{"Rx", "Tx"}."Tx" ("值(信号)")) -> ()  [unwired: 2 in, 2 out]
            n122 = flat-sequence {
              frame #0 {
                n123 = local write "successful ？"(FALSE ("successful ？")) -> ()
              }
              frame #1 {
                n124 = Wait (ms)(milliseconds to wait=u32 50 ("等待时间（毫秒）")) -> ()  [unwired: 1 out]
              }
            }
            n125 = To Variant(anything="Cycle 2") -> (Variant=w1107:variant)
            n126 = Bundle By Name(cluster=T27 {"Sender"="", "receiver"="", "message"="SendHead&Receive", "data"=variant} ("Communication message"), "message"="Send_Frame", "data"=w1107) -> (w1108:T27)
          }
          event "LIN_Schedule_Tab": Value Change {
            n127 = event-data() -> ()  [unwired: 1 in, 1 out]
            n128 = Bundle By Name(cluster=T27 {"Sender"="", "receiver"="", "message"="SendHead&Receive", "data"=variant} ("Communication message"), "message"="LIN_Schedule_Tab") -> (w1116:T27)
          }
          event "Clear": Value Change {
            n129 = event-data() -> ()  [unwired: 1 in, 1 out]
          }
          event "DLL_PATH", "Channel", "ALINId", "ALINDLC", "Rx/TX", "LIN_DATA", "Timeout", "async&sync", "Read Message Type", "LIN_Data.LIN_Set_Array", "LDF Path", "LDF loading channel", "BLF_Log_PATH", "Channels used", "REC_Channel": Value Change {
            # "Update data when control value changes"
            n130 = event-data() -> ()  [unwired: 1 in, 1 out]
            n131 = Bundle By Name(cluster=T20 {"ALINIdxchn"=0, "ALINId"=0, "ALINDLC"=0} ("LIN_Data.LIN_SendHead"), "ALINIdxchn"="Channel", "ALINId"="ALINId", "ALINDLC"="ALINDLC") -> (w1148:T20)
            n132 = Bundle By Name(cluster=w1150, "LIN_Data.Blf_Log.Blf_Log_PATH"="BLF_Log_PATH", "LIN_Data.LDF.LDF Path"="LDF Path", "LIN_Data.LDF.LDF loading channel"="LDF loading channel", "LIN_Data.DLL_PATH"="DLL_PATH", "LIN_Data.sync_sendTimeout"="Timeout", "LIN_Data.LIN_DATA"="LIN_DATA", "LIN_Data.Rx/TX"="Rx/TX", "LIN_Data.LIN_SendHead"=w1148, "LIN_Data.Read message type"="Read Message Type", "LIN_Data.Channels used"="Channels used", "LIN_Data.LIN_Set_Array"="LIN_Data.LIN_Set_Array", "LIN_Data.async&sync"="async&sync", "LIN_Data.REC_Channel"="REC_Channel") -> (w1143:T18)
            n133 = case shown="\"async\", 默认" "async&sync" {
              tunnel: [T17."Disabled and Grayed Out" ("禁用") T17."Enabled" ("禁用")] -> w1137
              frame "async", Default {
              }
              frame "sync" {
              }
            }
            n134 = To Variant(anything=w1143) -> (Variant=w1142:variant)
            n135 = property on="Timeout" class="DigNum (严格)"("DisabledEnum"=w1137) -> ()  [unwired: 2 in, 2 out]
            n136 = Bundle By Name(cluster=T27 {"Sender"="", "receiver"="", "message"="", "data"=variant} ("Communication message"), "message"="Config update", "data"=w1142) -> (w1144:T27)
          }
          event "Diagram shown": Value Change {
            n137 = event-data() -> ("NewVal"=w1154:bool)  [unwired: 1 in]
            n138 = To Variant(anything=w1154) -> (Variant=w1155:variant)
            n139 = Bundle By Name(cluster=T27 {"Sender"="", "receiver"="", "message"="", "data"=variant} ("Communication message"), "message"="Diagram shown", "data"=w1155) -> (w1156:T27)
          }
          event "Load_LDF": Value Change {
            n140 = event-data() -> ()  [unwired: 1 in, 1 out]
            n141 = Bundle By Name(cluster=T27 {"Sender"="", "receiver"="", "message"="", "data"=variant} ("Communication message"), "message"="Load_LDF") -> (w1163:T27)
          }
          event "Unload": Value Change {
            n142 = event-data() -> ()  [unwired: 1 in, 1 out]
            n143 = Bundle By Name(cluster=T27 {"Sender"="", "receiver"="", "message"="", "data"=variant} ("Communication message"), "message"="Unload") -> (w1168:T27)
          }
          event "Start Log": Value Change {
            n144 = event-data() -> ()  [unwired: 1 in, 1 out]
            n145 = Bundle By Name(cluster=T27 {"Sender"="", "receiver"="", "message"="", "data"=variant} ("Communication message"), "message"="Start Log") -> (w1174:T27)
          }
          event "Stop Log": Value Change {
            n146 = event-data() -> ()  [unwired: 1 in, 1 out]
            n147 = Bundle By Name(cluster=T27 {"Sender"="", "receiver"="", "message"="", "data"=variant} ("Communication message"), "message"="Stop Log") -> (w1180:T27)
          }
          event "Export", "Import": Value Change {
            # "Import or export configuration"
            n148 = event-data() -> ("CtlRef"=w1189:refnum<vi>)  [unwired: 1 in]
            n149 = property class="Bool"(reference=w1189) -> ("Label.Text"=w1186:string)  [unwired: 1 in, 2 out]
            n150 = Bundle By Name(cluster=T27 {"Sender"="", "receiver"="", "message"="", "data"=variant} ("Communication message"), "message"=w1186) -> (w1187:T27)
          }
          event User Event {
            # "Receive user events"
            n151 = event-data() -> ("Message"=w1198:string)  [unwired: 1 in]
            n152 = Equal?(x=w1198, y="Quit") -> (x = y?=w1196:bool)
          }
          event "Tree control": Mouse Up {
            n153 = event-data() -> ("CtlRef"=w1200:refnum<vi>)  [unwired: 1 in, 1 out]
            n154 = To Variant(anything=w1200) -> (Variant=w1202:variant)
            n155 = Bundle By Name(cluster=T27 {"Sender"="", "receiver"="", "message"="", "data"=variant} ("Communication message"), "message"="LDF_Define", "data"=w1202) -> (w1201:T27)
          }
          event Panel Close? {
            w1214 = TRUE ("放弃？")
            n156 = event-data() -> ()  [unwired: 1 in, 4 out]
            n157 = Bundle By Name(cluster=T27 {"Sender"="", "receiver"="", "message"="", "data"=variant} ("Communication message"), "message"="Quit") -> (w1209:T27)
            n158 = event-data("Discard?"=w1214) -> ()  [unwired: 1 in, 1 out]
          }
          event "STOP": Value Change {
            n159 = event-data() -> ()  [unwired: 1 in, 1 out]
          }
        }
        n160 = Unbundle By Name(w1041) -> ("message"=w1040:string)
        n161 = case shown="\"default\", 默认" w1040 {
          tunnel: w1044 -> [w1051 w1053]
          tunnel: w1042 -> [w1050 w1052]
          tunnel: w1041 -> [w1047 _]
          tunnel: [w1049 w1053] -> _
          tunnel: [w1048 w1052] -> _
          frame "default", Default {
            n162 = Enqueue Element(queue=w1051, element=w1047, error in (no error)=w1050) -> (queue out=w1049:refnum<queue>, error out=w1048:errorcluster)  [unwired: 1 in, 1 out]
          }
          frame "" {
          }
        }
      }
      n163 = while {
        tunnel: w94 -> [w185]
        tunnel: w93 -> [w184]
        tunnel: [w177] -> w81
        tunnel: [w176] -> w80
        shift-right: [w165] -> _
        shift-left: w84 -> [w173]
        tunnel: w86 -> [w170]
        tunnel: w85 -> [w169]
        tunnel: w82 -> [w168]
        stop <- w175 stop-if-true
        # "Processing"
        n164 = Dequeue Element(queue=w185, error in (no error)=w184) -> (queue out=w182:refnum<queue>, element=w172:T27, error out=w181:errorcluster)  [unwired: 1 in, 1 out]
        n165 = Unbundle By Name(w172) -> ("message"=w183:string, "data"=w178:variant)
        n166 = case shown="\"Connect\"" w183 {
          selector: w183 -> [_ _ _ w230 _ w305 _ _ _ _ _ _ _ _ _ _ _ _ _ _ _ _ _ _]
          tunnel: [w195 w199 w221 w238 w264 w314 w348 w363 w394 w424 w451 w476 w492 w543 w598 w618 w638 w650 w670 w687 w970 w987 w998 w1022] -> w180
          tunnel: w182 -> [w195 w199 w221 w238 w264 w314 w348 w369 w394 w424 w451 w476 w493 w544 w598 w618 w638 w650 w670 w687 w970 w987 w998 w1022]
          tunnel: w181 -> [w194 w198 w219 w237 w262 w313 w347 w362 w393 w423 w450 w475 w491 w548 w594 w617 w637 w649 w669 w686 w969 w986 w997 w1021]
          tunnel: [w194 w198 w219 w237 w262 w313 w347 w361 w393 w423 w450 w475 w490 w542 w593 w613 w637 w649 w669 w686 w969 w986 w997 w1021] -> w179
          tunnel: w178 -> [_ _ _ _ _ w306 _ w358 w386 _ _ _ w499 w545 _ _ w640 w643 _ w684 _ _ _ _]
          tunnel: [_ _ _ _ _ _ _ _ _ _ _ _ _ _ _ _ _ _ _ _ _ _ _ TRUE] -> w175
          tunnel: [w193 w197 w218 w229 w261 w310 w345 w366 w384 w422 w449 w465 w504 w551 w595 w616 w619 w642 w656 w674 w954 w975 w988 w1017] -> w167
          tunnel: w173 -> [w193 w197 w220 w236 w263 w312 w346 w368 w385 w418 w449 w465 w505 w549 w596 w609 w625 w648 w668 w674 w954 w976 w989 w1019]
          tunnel: [_ T27 {"Sender"="", "receiver"="", "message"="", "data"=variant} ("Communication message") w203 w227 _ w307 _ _ _ w414 _ _ w497 w539 _ _ _ _ _ _ _ _ _ _] -> w171
          tunnel: w172 -> [_ _ _ _ _ _ _ _ _ _ _ _ _ _ _ _ _ _ _ _ _ _ _ _]
          tunnel: w170 -> [_ _ _ _ _ _ _ _ _ _ _ _ w485 _ _ w612 w633 _ w658 _ w959 _ _ w1014]
          tunnel: w169 -> [_ _ _ _ _ _ _ _ _ _ _ _ w484 _ _ w611 w632 _ w657 _ w958 _ _ w1013]
          tunnel: w168 -> [_ _ _ _ _ _ _ _ _ _ _ _ _ _ _ _ _ _ _ _ _ _ _ w1006]
          frame "eee", Default {
          }
          frame "" {
          }
          frame "Init" {
            n167 = Unbundle By Name(w220) -> ("Communication message.Sender"=w214:string, "LIN_Data.DLL_PATH"=w202:path)
            n168 = call "initialize_lib_tsmaster.vi"("AppName"=w214, "Path input"=w202) -> ("error output"=w216:errorcluster, "Path output"=w215:path)  [unwired: 8 in]
            n169 = call "tsapp_disconnect.vi"("error in (no error)"=w216, "Path"=w215) -> ("error output"=w209:errorcluster, "retuen"=w213:i32, "Path output"=w210:path)  [unwired: 7 in]
            n170 = call "Device_Detection.vi"("error in (no error)"=w209, "Path"=w210) -> ("error out"=w201:errorcluster, "retuen"=w208:i32)  [unwired: 7 in, 1 out]
            n171 = Equal To 0?(x=w208) -> (x = 0?=w207:bool)
            n172 = Unbundle By Name(w201) -> ("status"=w200:bool)
            n173 = Equal To 0?(x=w213) -> (x = 0?=w212:bool)
            n174 = Not(x=w200) -> (.not. x?=w206:bool)
            n175 = Compound Arithmetic op=AND(w212, w207, w206) -> (w217:bool)
            n176 = case shown="假" w217 {
              tunnel: ["Config fail" ("消息") "Config Successful  " ("消息")] -> w211
              frame False {
              }
              frame True {
              }
            }
            n177 = call "Log.vi"("Data"=w211) -> ()  [unwired: 3 in]
            n178 = Bundle By Name(cluster=w220, "error in"=w201) -> (w218:T18)
            n179 = Bundle By Name(cluster=T27 {"Sender"="", "receiver"="", "message"="", "data"=variant} ("Communication message"), "message"="Channel_Count") -> (w203:T27)
          }
          frame "Channel_Count" {
            n180 = Unbundle By Name(w236) -> ("Communication message.Sender"=w224:string, "LIN_Data.DLL_PATH"=w235:path, "LIN_Data.Channels used"=w234:u16, "AsynCall?"=w226:bool)
            n181 = Concatenate Strings(w224, w230) -> (w225:string)
            n182 = call "tsapp_set_lin_channel_count.vi"("Aount"=w234, "Path"=w235) -> ("error out"=w231:errorcluster, "return"=w232:i32, "Path output"=w233:path)  [unwired: 7 in]
            n183 = call "error_display.vi"("error in"=w231, "Action name"=w225, "return"=w232, "DLL path"=w233) -> ("error out"=w228:errorcluster)  [unwired: 6 in, 1 out]
            n184 = Bundle By Name(cluster=w236, "error in"=w228) -> (w229:T18)
            n185 = case shown="假" w226 {
              tunnel: [w239 T27 {"Sender"="", "receiver"="", "message"="", "data"=variant} ("Communication message")] -> w227
              frame False {
                n186 = Bundle By Name(cluster=T27 {"Sender"="", "receiver"="", "message"="", "data"=variant} ("Communication message"), "message"="Mapping") -> (w239:T27)
              }
              frame True {
              }
            }
          }
          frame "Mapping" {
            n187 = Unbundle By Name(w263) -> ("Communication message.receiver"=w246:string, "Communication message.Sender"=w245:string, "LIN_Data.DLL_PATH"=w251:path, "LIN_Data.LIN_Set_Array"=w250:T9[], "AsynCall?"=w248:bool)
            n188 = Select(t=w246, s=w248, f=w245) -> (s? t:f=w247:string)
            n189 = case shown="真" "TS_Mapping" {
              tunnel: [w274 w287] -> w257
              tunnel: w247 -> [w271 _]
              tunnel: w250 -> [w270 _]
              tunnel: [w269 w292] -> w256
              tunnel: [w268 w292] -> w255
              tunnel: [TRUE w292] -> w254
              tunnel: w251 -> [w267 w291]
              tunnel: "CH_Mapping" -> [_ w290]
              tunnel: [TRUE w285] -> w243
              frame False {
                n190 = for {
                  tunnel: w267 -> [w283]
                  tunnel: [w279] -> w273 mode=indexing
                  tunnel: [w278] -> w272 mode=indexing
                  tunnel: w271 -> [w277]
                  shift-right: [w282] -> w274
                  shift-left: _ -> [w284]
                  tunnel: w270 -> [w276] mode=indexing
                  n191 = Unbundle By Name(w276) -> ("Set"=w275:T10)
                  n192 = call "TSLIN_SetData.vi"("Error in"=w284, "AppName"=w277, "Set"=w275, "Path"=w283) -> ("Error out"=w282:errorcluster, "mapping_return"=w280:i32, "config_baud_return"=w281:i32)  [unwired: 4 in, 1 out]
                  n193 = Equal To 0?(x=w281) -> (x = 0?=w279:bool)
                  n194 = Equal To 0?(x=w280) -> (x = 0?=w278:bool)
                }
                n195 = And Array Elements(Boolean array=w272) -> (logical AND=w268:bool)
                n196 = And Array Elements(Boolean array=w273) -> (logical AND=w269:bool)
              }
              frame True {
                n197 = call "tsapp_show_hardware_configuration_window.vi"("路径输入"=w291) -> ("error out"=w288:errorcluster, "function return"=w293:i32, "路径输出"=w289:path)  [unwired: 8 in]
                n198 = Equal To 0?(x=w293) -> (x = 0?=w292:bool)
                n199 = case shown="真" w290 {
                  tunnel: w289 -> [w295 w300]
                  tunnel: w288 -> [w294 w298]
                  tunnel: [w295 w299] -> _
                  tunnel: [_ w296] -> w286
                  tunnel: [w294 w297] -> w287
                  frame False {
                  }
                  frame True {
                    n200 = call "tsapp_show_channel_mapping_window.vi"("error in (no error)"=w298, "路径输入"=w300) -> ("error out"=w297:errorcluster, "function return"=w296:i32, "路径输出"=w299:path)  [unwired: 7 in]
                  }
                }
                n201 = Equal To 0?(x=w286) -> (x = 0?=w285:bool)
              }
            }
            n202 = Unbundle By Name(w257) -> ("status"=w260:bool)
            n203 = Not(x=w260) -> (.not. x?=w259:bool)
            n204 = Compound Arithmetic op=AND(w243, w254, w256, w255, w259) -> (w258:bool)
            n205 = case shown="真" w258 {
              tunnel: ["Mapping fail" ("消息") "Mapping Successful  " ("消息")] -> w253
              frame False {
              }
              frame True {
              }
            }
            n206 = Bundle By Name(cluster=w263, "error in"=w257) -> (w261:T18)
            n207 = Concatenate Strings(w245, w253) -> (w249:string)
            n208 = call "Log.vi"("Data"=w249) -> ()  [unwired: 3 in]
          }
          frame "Connect" {
            n209 = Unbundle By Name(w312) -> ("LIN_Data.DLL_PATH"=w311:path, "AsynCall?"=w303:bool)
            n210 = case shown="真" w303 {
              tunnel: w311 -> [w329 _]
              tunnel: [w323 w331] -> w304
              tunnel: [w318 w330] -> w309
              tunnel: w306 -> [_ w333]
              tunnel: w305 -> [w321 _]
              frame False {
                n211 = call "tsapp_connect.vi"("Path"=w329) -> ("error out"=w324:errorcluster, "retuen"=w322:i32, "Path output"=w325:path)  [unwired: 8 in]
                n212 = Equal To 0?(x=w322) -> (x = 0?=w326:bool)
                n213 = call "tsfifo_enable_receive_fifo.vi"("error in (no error)"=w324, "Path"=w325) -> ("error out"=w319:errorcluster, "Path output"=w320:path)  [unwired: 8 in]
                n214 = Unbundle By Name(w319) -> ("status"=w328:bool)
                n215 = call "error_display.vi"("error in"=w319, "Action name"=w321, "return"=w322, "DLL path"=w320) -> ("error out"=w318:errorcluster)  [unwired: 6 in, 1 out]
                n216 = Not(x=w328) -> (.not. x?=w327:bool)
                n217 = Compound Arithmetic op=AND(w327, w326) -> (w323:bool)
              }
              frame True {
                n218 = Variant To Data(type=FALSE, Variant=w333) -> (data=w331:bool, error out=w330:errorcluster)  [unwired: 1 in]
              }
            }
            "Connect ?" <- w304
            n219 = Bundle By Name(cluster=w312, "error in"=w309) -> (w310:T18)
            n220 = case shown="真" w304 {
              tunnel: ["Conncet  fail" ("消息") "Conncet  Successful" ("消息")] -> w308
              frame False {
              }
              frame True {
              }
            }
            n221 = call "Log.vi"("Data"=w308) -> ()  [unwired: 3 in]
            n222 = case shown="真" w304 {
              tunnel: [_ w315] -> w307
              frame False {
              }
              frame True {
                n223 = Bundle By Name(cluster=T27 {"Sender"="", "receiver"="", "message"="", "data"=variant} ("Communication message"), "message"="Set Node") -> (w315:T27)
              }
            }
          }
          frame "Set Node" {
            n224 = Unbundle By Name(w346) -> ("LIN_Data.DLL_PATH"=w336:path, "LIN_Data.LIN_Set_Array"=w341:T9[])
            n225 = for {
              tunnel: w341 -> [w353] mode=indexing
              tunnel: [w350] -> w340 mode=indexing
              tunnel: w336 -> [w355]
              tunnel: [w354] -> w337
              n226 = Unbundle By Name(w353) -> ("Set.AAppChannel"=w352:i32, "Set_node_funtiontype"=w351:i32)
              n227 = call "tslin_set_node_funtiontype.vi"("set_node_funtiontype"=w351, "AAppChannel"=w352, "path"=w355) -> ("错误输出"=w354:errorcluster, "return"=w349:i32)  [unwired: 6 in, 1 out]
              n228 = Equal To 0?(x=w349) -> (x = 0?=w350:bool)
            }
            n229 = And Array Elements(Boolean array=w340) -> (logical AND=w339:bool)
            n230 = Unbundle By Name(w337) -> ("status"=w343:bool)
            n231 = Not(x=w343) -> (.not. x?=w342:bool)
            n232 = Compound Arithmetic op=AND(w339, w342) -> (w344:bool)
            n233 = case shown="假" w344 {
              tunnel: ["Set Node  fail" ("消息") "Set Node  Successful" ("消息")] -> w338
              frame False {
              }
              frame True {
              }
            }
            n234 = Bundle By Name(cluster=w346, "error in"=w337) -> (w345:T18)
            n235 = call "Log.vi"("Data"=w338) -> ()  [unwired: 3 in]
          }
          frame "Disconnect" {
            n236 = Unbundle By Name(w368) -> ("LIN_Data.DLL_PATH"=w367:path, "AsynCall?"=w359:bool)
            n237 = case shown="真" w359 {
              tunnel: w367 -> [w376 _]
              tunnel: [w374 w377] -> w365
              tunnel: [w372 w378] -> w364
              tunnel: w358 -> [_ w380]
              frame False {
                n238 = call "tsapp_disconnect.vi"("Path"=w376) -> ("error output"=w372:errorcluster, "retuen"=w375:i32)  [unwired: 8 in, 1 out]
                n239 = Equal To 0?(x=w375) -> (x = 0?=w370:bool)
                n240 = Unbundle By Name(w372) -> ("status"=w373:bool)
                n241 = Not(x=w373) -> (.not. x?=w371:bool)
                n242 = And(x=w371, y=w370) -> (x .and. y?=w374:bool)
              }
              frame True {
                n243 = Variant To Data(type=FALSE, Variant=w380) -> (data=w377:bool, error out=w378:errorcluster)  [unwired: 1 in]
              }
            }
            n244 = Flush Queue(queue=w369, error in (no error)=w362) -> (queue out=w363:refnum<queue>, error out=w361:errorcluster)  [unwired: 1 out]
            n245 = Bundle By Name(cluster=w368, "error in"=w364) -> (w366:T18)
            n246 = case shown="假" w365 {
              tunnel: ["Disconncet  fail" ("消息") "Disconncet  Successful" ("消息")] -> w360
              frame False {
              }
              frame True {
                n247 = local write "Connect ?"(FALSE ("Connect ?")) -> ()
              }
            }
            n248 = call "Log.vi"("Data"=w360) -> ()  [unwired: 3 in]
          }
          frame "DIS_REC" {
            n249 = Variant To Data(type=FALSE, Variant=w386) -> (data=w391:bool, error out=w389:errorcluster)  [unwired: 1 in]
            n250 = Unbundle By Name(w385) -> ("LIN_Data.DLL_PATH"=w390:path, "LIN_Data.REC_Channel"=w387:i32)
            n251 = case shown="真" w391 {
              tunnel: w390 -> [w395 w404]
              tunnel: w389 -> [w397 w412]
              tunnel: [w398 w400] -> w388
              tunnel: w387 -> [_ w402]
              frame False {
                n252 = call "tsfifo_enable_receive_fifo.vi"("error in (no error)"=w397, "Path"=w395) -> ("error out"=w398:errorcluster)  [unwired: 8 in, 1 out]
                n253 = call "Log.vi"("Data"="EN_REC") -> ()  [unwired: 3 in]
              }
              frame True {
                w410 = "clear_receive_buffers Successful"  # clear_receive_buffers Successful
                n254 = call "tsfifo_disable_receive_fifo.vi"("error in (no error)"=w412, "Path"=w404) -> ("error out"=w401:errorcluster, "Path output"=w403:path)  [unwired: 8 in]
                n255 = call "tsfifo_clear_lin_receive_buffers.vi"("error in (no error)"=w401, "AIdxChn"=w402, "路径输入"=w403) -> ("error out"=w400:errorcluster, "return"=w399:i32)  [unwired: 6 in, 1 out]
                n256 = Equal To 0?(x=w399) -> (x = 0?=w411:bool)
                n257 = Select(t=w410, s=w411, f="clear_receive_buffers Fail") -> (s? t:f=w408:string)
                n258 = Concatenate Strings("DIS_REC" ("string"), "\r", w408) -> (w407:string)
                n259 = call "Log.vi"("Data"=w407) -> ()  [unwired: 3 in]
              }
            }
            n260 = Bundle By Name(cluster=w385, "error in"=w388) -> (w384:T18)
          }
          frame "Import" {
            n261 = Read from Binary File(5:w418, 7:"Please select a configuration file" ("对话框窗口（打开现有文件）")) -> (0:w421:errorcluster, 1:w419:bool, 2:w420:T18)  [unwired: 4 in, 1 out]
            n262 = case shown="无错误" w421 {
              selector: w421 -> [_ w442]
              tunnel: w420 -> [w428 _]
              tunnel: w419 -> [w430 _]
              tunnel: w418 -> [w429 w445]
              tunnel: [w427 w445] -> w422
              tunnel: [w426 w439] -> w416
              tunnel: [w425 _] -> w413
              frame No Error {
                n263 = case shown="假" w430 {
                  tunnel: w429 -> [w437 w438]
                  tunnel: w428 -> [w436 _]
                  tunnel: [w434 w438] -> w427
                  tunnel: [w432 _] -> w426
                  tunnel: ["update" ("message") _] -> w425
                  frame False {
                    w432 = "Import successful" ("消息")
                    n264 = Unbundle By Name(w436) -> ("LIN_Data"=w435:T19)
                    n265 = Bundle By Name(cluster=w437, "LIN_Data"=w435) -> (w434:T18)
                    n266 = One Button Dialog(message=w432, button name ("OK")="OK" ("按钮名称（“确定”）")) -> ()  [unwired: 1 out]
                  }
                  frame True {
                  }
                }
              }
              frame Error {
                n267 = call <vilib>:"Clear Errors.vi"("error in (no error)"=w442) -> ()  [unwired: 5 in, 2 out]
                n268 = Unbundle By Name(w442) -> ("source"=w443:string)
                n269 = Concatenate Strings("Import Fail" ("消息"), "\r", w443) -> (w439:string)
                n270 = One Button Dialog(message=w439, button name ("OK")="OK" ("按钮名称（“确定”）")) -> ()  [unwired: 1 out]
              }
            }
            n271 = call "Log.vi"("Data"=w416) -> ()  [unwired: 3 in]
            n272 = Bundle By Name(cluster=T27 {"Sender"="", "receiver"="", "message"="", "data"=variant} ("Communication message"), "message"=w413) -> (w414:T27)
          }
          frame "Export" {
            n273 = Write to Binary File(data=w449, 7:"Please edit the configuration name " ("提示（选择或输入文件路径）")) -> (error out=w447:errorcluster)  [unwired: 4 in, 2 out]
            n274 = case shown="无错误" w447 {
              selector: w447 -> [_ w455]
              tunnel: [w452 w454] -> w446
              frame No Error {
                w452 = "Export successful" ("消息")
                n275 = One Button Dialog(message=w452, button name ("OK")="OK" ("按钮名称（“确定”）")) -> ()  [unwired: 1 out]
              }
              frame Error {
                n276 = Unbundle By Name(w455) -> ("source"=w457:string)
                n277 = Concatenate Strings("Export Fail" ("消息"), "\r", w457) -> (w454:string)
                n278 = call <vilib>:"Clear Errors.vi"("error in (no error)"=w455) -> ()  [unwired: 5 in, 2 out]
                n279 = One Button Dialog(message=w454, button name ("OK")="OK" ("按钮名称（“确定”）")) -> ()  [unwired: 1 out]
              }
            }
            n280 = call "Log.vi"("Data"=w446) -> ()  [unwired: 3 in]
          }
          frame "update" {
            n281 = Unbundle By Name(w465) -> ("LIN_Data.DLL_PATH"=w474:path, "LIN_Data.Channels used"=w473:u16, "LIN_Data.Rx/TX"=w472:enum16{"Rx", "Tx"}, "LIN_Data.Read message type"=w471:T14, "LIN_Data.async&sync"=w470:enum16{"async", "sync"}, "LIN_Data.sync_sendTimeout"=w469:u16, "LIN_Data.LIN_SendHead.ALINIdxchn"=w468:u8, "LIN_Data.LIN_SendHead.ALINId"=w467:u32, "LIN_Data.LIN_SendHead.ALINDLC"=w466:u32)
            n282 = local write "LDF Path"(w474) -> ()
            n283 = local write "Channels used"(w473) -> ()
            n284 = local write "Rx/TX"(w472) -> ()
            n285 = local write "Read Message Type"(w471) -> ()
            n286 = local write "async&sync"(w470) -> ()
            n287 = local write "Timeout"(w469) -> ()
            n288 = local write "Channel"(w468) -> ()
            n289 = local write "ALINId"(w467) -> ()
            n290 = local write "ALINDLC"(w466) -> ()
            n291 = Unbundle By Name(w465) -> ("LIN_Data.LIN_DATA"=w464:T13, "LIN_Data.LIN_Set_Array"=w463:T9[], "LIN_Data.LDF.LDF Path"=w462:path, "LIN_Data.LDF.LDF loading channel"=w461:i32, "LIN_Data.Blf_Log.Blf_Log_PATH"=w460:path)
            n292 = local write "LIN_DATA"(w464) -> ()
            n293 = local write "LIN_Data.LIN_Set_Array"(w463) -> ()
            n294 = local write "LDF Path"(w462) -> ()
            n295 = local write "LDF loading channel"(w461) -> ()
            n296 = local write "BLF_Log_PATH"(w460) -> ()
          }
          frame "SendHead&Receive" {
            n297 = Variant To Data(type=FALSE, Variant=w499) -> (data=w495:bool, error out=w496:errorcluster)  [unwired: 1 in]
            n298 = case shown="无错误" w496 {
              selector: w496 -> [_ w521]
              tunnel: w495 -> [w506 _]
              tunnel: [w506 FALSE] -> w494
              tunnel: w493 -> [w510 w520]
              tunnel: w491 -> [w509 w519]
              tunnel: [w508 w518] -> w492
              tunnel: [w507 w517] -> w490
              frame No Error {
                n299 = case shown="假" w506 {
                  tunnel: w510 -> [w514 w516]
                  tunnel: w509 -> [w513 w515]
                  tunnel: [w512 w516] -> w508
                  tunnel: [w511 w515] -> w507
                  frame False {
                    n300 = Flush Queue(queue=w514, error in (no error)=w513) -> (queue out=w512:refnum<queue>, error out=w511:errorcluster)  [unwired: 1 out]
                  }
                  frame True {
                  }
                }
              }
              frame Error {
                n301 = call <vilib>:"Clear Errors.vi"("error in (no error)"=w521) -> ()  [unwired: 5 in, 2 out]
                n302 = Flush Queue(queue=w520, error in (no error)=w519) -> (queue out=w518:refnum<queue>, error out=w517:errorcluster)  [unwired: 1 out]
              }
            }
            n303 = Wait (ms)(milliseconds to wait=u32 100 ("等待时间（毫秒）")) -> ()  [unwired: 1 out]
            n304 = Unbundle By Name(w505) -> ("LIN_Data.DLL_PATH"=w503:path, "LIN_Data.LIN_SendHead.ALINIdxchn"=w486:u8, "LIN_Data.LIN_SendHead.ALINId"=w487:u32, "LIN_Data.LIN_SendHead.ALINDLC"=w502:u32)
            n305 = call "tsapp_transmit_header_and_receive_msg.vi"("ATimeoutMs"="ATimeoutMs", "ADLC"=w502, "AIdentifier"=w487, "AChn"=w486, "Path"=w503) -> ("错误输出"=w488:errorcluster, "return"=w489:i32, "ALINData"=w500:T16)  [unwired: 2 in, 1 out]
            n306 = Equal To 0?(x=w489) -> (x = 0?=→"Successful ?":bool)
            n307 = Build Array(w500) -> (w481:T16[])
            n308 = To Variant(anything="SendHead&Receive" ("Sender")) -> (Variant=w479:variant)
            n309 = Bundle By Name(cluster=T26 {"Sender"="", "receiver"="", "message"="", "data"=variant, "LIN Data array"=[]} ("Communication message"), "LIN Data array"=w481, "data"=w479) -> (w482:T26)
            n310 = Enqueue Element(queue=w485, element=w482, error in (no error)=w484) -> ()  [unwired: 1 in, 3 out]
            n311 = case shown="真" w494 {
              tunnel: [T27 {"Sender"="", "receiver"="", "message"="", "data"=variant} ("Communication message") w527] -> w497
              frame False {
              }
              frame True {
                n312 = To Variant(anything=TRUE) -> (Variant=w525:variant)
                n313 = Bundle By Name(cluster=T27 {"Sender"="", "receiver"="", "message"="", "data"=variant} ("Communication message"), "message"="SendHead&Receive", "data"=w525) -> (w527:T27)
              }
            }
            n314 = Bundle By Name(cluster=w505, "error in"=w488) -> (w504:T18)
          }
          frame "Send_Frame" {
            n315 = Unbundle By Name(w549) -> ("LIN_Data.async&sync"=w537:enum16{"async", "sync"}, "LIN_Data.sync_sendTimeout"=w538:u16, "LIN_Data.DLL_PATH"=w557:path, "LIN_Data.LIN_SendHead.ALINIdxchn"=w531:u8, "LIN_Data.Rx/TX"=w547:enum16{"Rx", "Tx"}, "LIN_Data.LIN_SendHead.ALINDLC"=w554:u32, "LIN_Data.LIN_SendHead.ALINId"=w553:u32, "LIN_Data.LIN_DATA"=w552:T13, "LIN_Data.LIN_Set_Array"=w532:T9[])
            n316 = Wait (ms)(milliseconds to wait=u32 100 ("等待时间（毫秒）")) -> ()  [unwired: 1 out]
            n317 = Variant To Data(type=FALSE, Variant=w545) -> (data=w541:bool, error out=w533:errorcluster)  [unwired: 1 in]
            n318 = Index Array(array=w532, index=w531) -> (element=w530:T9)
            n319 = Unbundle By Name(w530) -> ("Set_node_funtiontype"=w529:i32)
            n320 = Bundle By Name(cluster=T23 {"Channel"=0, "Rx/TX"=enum."Rx", "Set_node_funtiontype"=0, "DLC"=0, "ID"=0, "FDatas"={"value0"=0, "value 1"=0, "value 2"=0, "value 3"=0, "value 4"=0, "value 5"=0, "value 6"=0, "value 7"=0}} ("LIN_Transmit"), "Channel"=w531, "Rx/TX"=w547, "Set_node_funtiontype"=w529, "DLC"=w554, "ID"=w553, "FDatas"=w552) -> (w555:T23)
            n321 = case shown="\"async\", 默认" w537 {
              tunnel: w557 -> [w563 w568]
              tunnel: w555 -> [w562 w570]
              tunnel: [w561 w567] -> w550
              tunnel: [w560 w569] -> _
              tunnel: w548 -> [w559 w565]
              tunnel: [w558 w566] -> w536
              tunnel: w538 -> [_ w564]
              frame "async", Default {
                n322 = call "tsapp_transmit_lin_async.vi"("error in (no error)"=w559, "LIN_Transmit"=w562, "Path"=w563) -> ("error out"=w558:errorcluster, "return"=w561:i32, "Path output"=w560:path)  [unwired: 6 in]
              }
              frame "sync" {
                n323 = call "tsapp_transmit_lin_sync.vi"("错误输入（无错误）"=w565, "ATimeoutMS"=w564, "LIN_Transmit"=w570, "路径输入"=w568) -> ("错误输出"=w566:errorcluster, "return"=w567:i32, "路径输出"=w569:path)  [unwired: 5 in]
              }
            }
            n324 = Equal To 0?(x=w550) -> (x = 0?=→"successful ？":bool)
            n325 = case shown="无错误" w533 {
              selector: w533 -> [w577 w591]
              tunnel: w541 -> [w578 _]
              tunnel: [w578 FALSE] -> w540
              tunnel: w544 -> [w581 w590]
              tunnel: [w580 w589] -> w543
              tunnel: [w579 w588] -> w542
              frame No Error {
                n326 = case shown="假" w578 {
                  tunnel: w581 -> [w585 w587]
                  tunnel: [w584 w587] -> w580
                  tunnel: [w583 w586] -> w579
                  tunnel: w577 -> [w582 w586]
                  frame False {
                    n327 = Flush Queue(queue=w585, error in (no error)=w582) -> (queue out=w584:refnum<queue>, error out=w583:errorcluster)  [unwired: 1 out]
                  }
                  frame True {
                  }
                }
              }
              frame Error {
                n328 = call <vilib>:"Clear Errors.vi"("error in (no error)"=w591) -> ()  [unwired: 5 in, 2 out]
                n329 = Flush Queue(queue=w590) -> (queue out=w589:refnum<queue>, error out=w588:errorcluster)  [unwired: 1 in, 1 out]
              }
            }
            n330 = case shown="真" w540 {
              tunnel: [T27 {"Sender"="", "receiver"="", "message"="", "data"=variant} ("Communication message") w575] -> w539
              frame False {
              }
              frame True {
                n331 = To Variant(anything=TRUE) -> (Variant=w573:variant)
                n332 = Bundle By Name(cluster=T27 {"Sender"="", "receiver"="", "message"="", "data"=variant} ("Communication message"), "message"="Send_Frame", "data"=w573) -> (w575:T27)
              }
            }
            n333 = Bundle By Name(cluster=w549, "error in"=w536) -> (w551:T18)
          }
          frame "LIN_Schedule_Tab" {
            n334 = call "TSLIN_LIN_Schedule_Tab.vi"("错误输入（无错误）"=w594, "Data"=w596, "Sender"="LIN_Schedule_Tab") -> ("错误输出"=w593:errorcluster, "Data out"=w595:T18)  [unwired: 7 in]
          }
          frame "Clear" {
            n335 = Bundle By Name(cluster=T26 {"Sender"="", "receiver"="", "message"="", "data"=variant, "LIN Data array"=[]} ("Communication message"), "message"="Clear") -> (w599:T26)
            n336 = local read "REC_Channel"() -> (w607:i32)
            n337 = Unbundle By Name(w609) -> ("LIN_Data.DLL_PATH"=w608:path)
            n338 = property on="LIN_Data_0" class="MCListbox (严格)"(error in=w617, "ItemNames"=string[][] [] ("项名")) -> (error out=w613:errorcluster)  [unwired: 1 in, 1 out]
            n339 = Enqueue Element(queue=w612, element=w599, error in (no error)=w611) -> ()  [unwired: 1 in, 3 out]
            n340 = call "tsfifo_clear_lin_receive_buffers.vi"("AIdxChn"=w607, "路径输入"=w608) -> ("error out"=w606:errorcluster, "return"=w604:i32)  [unwired: 7 in, 1 out]
            n341 = Equal To 0?(x=w604) -> (x = 0?=w605:bool)
            n342 = Bundle By Name(cluster=w609, "LIN Data array"=T16[] [], "error in"=w606) -> (w616:T18)
            n343 = Select(t="Clear buffer Successful", s=w605, f="Clear buffer Fail") -> (s? t:f=w601:string)
            n344 = call "Log.vi"("Data"=w601) -> ()  [unwired: 3 in]
          }
          frame "Config update" {
            n345 = Unbundle By Name(w625) -> ("Communication message.Sender"=w624:string)
            n346 = Variant To Data(type=w625, Variant=w640) -> (data=w639:T18, error out=w634:errorcluster)  [unwired: 1 in]
            n347 = Unbundle By Name(w639) -> ("LIN_Data"=w628:T19)
            n348 = Bundle By Name(cluster=w625, "LIN_Data"=w628) -> (w626:T18)
            n349 = Current VI's Path() -> (path=w623:path)
            n350 = Strip Path(path=w623) -> (stripped path=w622:path)  [unwired: 1 out]
            n351 = To Variant(anything=w626) -> (Variant=w629:variant)
            n352 = Bundle By Name(cluster=T26 {"Sender"="", "receiver"="", "message"="", "data"=variant, "LIN Data array"=[]} ("Communication message"), "data"=w629, "message"="Config update") -> (w630:T26)
            n353 = Build Path(base path=w622, name or relative path="data") -> (appended path=w620:path)
            n354 = call "TSLIN_Configuration_Save.vi"("path"=w620, "error in (no error)"=w634, "Config Name"=w624, "Read/Write"=enum16{"Read", "Write"}."Write", "LIN_Data"=w628) -> ("error in (no error) 2"=w635:errorcluster)  [unwired: 4 in, 2 out]
            n355 = Enqueue Element(queue=w633, element=w630, error in (no error)=w632) -> ()  [unwired: 1 in, 3 out]
            n356 = Bundle By Name(cluster=w626, "error in"=w635) -> (w619:T18)
          }
          frame "Diagram shown" {
            n357 = Variant To Data(type=FALSE, Variant=w643) -> (data=w645:bool, error out=w644:errorcluster)  [unwired: 1 in]
            n358 = control-ref of="本VI"() -> (w647:refnum<vi>)
            n359 = property on="Property Node" class="VI"(reference=w647, error in=w644, "BDWin.Open"=w645) -> (error out=w641:errorcluster)  [unwired: 1 out]
            n360 = Bundle By Name(cluster=w648, "error in"=w641) -> (w642:T18)
          }
          frame "Load_LDF" {
            n361 = Unbundle By Name(w668) -> ("DataBase_array"=w651:T24, "LIN_Data.DLL_PATH"=w665:path, "LIN_Data.LDF.LDF Path"=w664:path, "LIN_Data.LDF.LDF loading channel"=w667:i32)
            n362 = Build Array(w667) -> (w666:i32[])
            n363 = call "LIN_LDF_Load.vi"("DataBase_array"=w651, "Channels"=w666, "LDF Path"=w664, "DLL_PATH"=w665) -> ("error out"=w662:errorcluster, "result"=w653:bool)  [unwired: 6 in]
            "Laod LDF Successful?" <- w653
            n364 = control-ref of="Tree control"() -> (w663:refnum<vi>)
            n365 = call "LIN_DBTableToTree.vi"("error in (no error)"=w662, "DataBase_array"=w651, "reference"=w663) -> ("error out"=w661:errorcluster)  [unwired: 8 in]
            n366 = Bundle By Name(cluster=w668, "error in"=w661) -> (w656:T18)
            n367 = case shown="真" w653 {
              tunnel: ["Load_LDF fail " ("消息") "Load_LDF successful " ("消息")] -> w652
              frame False {
              }
              frame True {
              }
            }
            n368 = To Variant(anything=w656) -> (Variant=w659:variant)
            n369 = Bundle By Name(cluster=T26 {"Sender"="", "receiver"="", "message"="", "data"=variant, "LIN Data array"=[]} ("Communication message"), "message"="Config update" ("Communication message.message"), "data"=w659) -> (w654:T26)
            n370 = call "Log.vi"("Data"=w652) -> ()  [unwired: 3 in]
            n371 = One Button Dialog(message=w652) -> ()  [unwired: 1 in, 1 out]
            n372 = Enqueue Element(queue=w658, element=w654, error in (no error)=w657) -> ()  [unwired: 1 in, 3 out]
          }
          frame "LDF_Define" {
            n373 = Variant To Data(type=refnum<vi> refnum ("CtlRef"), Variant=w684) -> (data=w681:refnum<vi>)  [unwired: 1 in, 1 out]
            n374 = property class="Tree (严格)"(reference=w681) -> (reference out=w683:refnum<vi>, error out=w682:errorcluster, "Value"=w675:string)  [unwired: 1 in]
            n375 = Unbundle By Name(w674) -> ("DataBase_array"=w673:T24)
            n376 = invoke class="Tree (严格)" method="Navigate Tree.Get Parent"(reference=w683, error in=w682, "tag"=w675) -> (reference out=w677:refnum<vi>, error out=w678:errorcluster, "Navigate Tree:Get Parent"=w676:string)  [unwired: 1 in, 1 out]
            n377 = xnode "匹配正则表达式"("输入字符串"=w676, "正则表达式"="_[0-9]+$" ("regular expression")) -> ("匹配之前"=w679:string)  [unwired: 4 in, 4 out]
            n378 = case shown="默认" w679 {
              tunnel: w678 -> [w695 _]
              tunnel: w677 -> [w694 _]
              tunnel: w676 -> [w691 _]
              tunnel: w673 -> [w688 w712]
              tunnel: w675 -> [w689 w713]
              frame Default {
                n379 = invoke class="Tree (严格)" method="Navigate Tree.Get Parent"(reference=w694, error in=w695, "tag"=w691) -> (error out=w696:errorcluster, "Navigate Tree:Get Parent"=w692:string)  [unwired: 1 in, 2 out]
                n380 = call <vilib>:"Clear Errors.vi"("error in (no error)"=w696) -> ()  [unwired: 5 in, 2 out]
                n381 = Equal?(x=w692, y="Messages") -> (x = y?=w690:bool)
                n382 = case shown="真" w690 {
                  tunnel: w689 -> [_ w698]
                  tunnel: w688 -> [_ w697]
                  frame False {
                  }
                  frame True {
                    n383 = control-ref of="Signal Table"() -> (w706:refnum<vi>)
                    n384 = property on="Property Node" class="Tbl (严格)"(reference=w706) -> (reference out=w702:refnum<vi>, error out=w700:errorcluster, "Value"=w704:string[][])  [unwired: 1 in]
                    n385 = call "LIN_Match_Signal.vi"("DataBase_array"=w697, "Signal"=w698) -> ("TDBSignalProperties"=w703:T5)  [unwired: 9 in]
                    n386 = call "LIN_Signal analysis.vi"("TDBSignalProperties"=w703, "Value in"=w704) -> ("Value out"=w699:string[][])  [unwired: 9 in]
                    n387 = property on="Property Node" class="Tbl (严格)"(reference=w702, error in=w700, "Value"=w699) -> ()  [unwired: 2 out]
                    n388 = control-ref of="LDF Tab"() -> (w705:refnum<vi>)
                    n389 = property on="Property Node" class="TabCtl (严格)"(reference=w705, "Value"=enum32{"Message", "Signal"}."Signal" ("Tab Control 2")) -> ()  [unwired: 1 in, 2 out]
                  }
                }
              }
              frame "Messages", "RX Message", "TX Message" {
                n390 = control-ref of="Message Table"() -> (w717:refnum<vi>)
                n391 = property on="Property Node" class="Tbl (严格)"(reference=w717) -> (reference out=w707:refnum<vi>, "Value"=w709:string[][])  [unwired: 1 in, 1 out]
                n392 = xnode "匹配正则表达式"("输入字符串"=w713, "正则表达式"="_[0-9]+$" ("regular expression")) -> ("匹配之前"=w711:string)  [unwired: 4 in, 4 out]
                n393 = call "LIN_Match_Message.vi"("DataBase_array"=w712, "Message"=w711) -> ("Frame"=w710:T28)  [unwired: 9 in]
                n394 = call "LIN_Message analysis.vi"("Frame"=w710, "Value in"=w709) -> ("Value out"=w708:string[][])  [unwired: 9 in]
                n395 = control-ref of="LDF Tab"() -> (w715:refnum<vi>)
                n396 = property on="Property Node" class="Tbl (严格)"(reference=w707, "Value"=w708) -> ()  [unwired: 1 in, 2 out]
                n397 = property on="Property Node" class="TabCtl (严格)"(reference=w715, "Value"=enum32{"Message", "Signal"}."Message" ("Tab Control 2")) -> ()  [unwired: 1 in, 2 out]
              }
            }
          }
          frame "Unload" {
            n398 = Unbundle By Name(w954) -> ("LIN_Data.DLL_PATH"=w968:path)
            n399 = call "tsdb_unload_lin_dbs.vi"("路径输入"=w968) -> ("error out"=w967:errorcluster, "function return"=w965:i32)  [unwired: 8 in, 1 out]
            n400 = Unbundle By Name(w967) -> ("status"=w966:bool)
            n401 = Equal To 0?(x=w965) -> (x = 0?=w964:bool)
            n402 = Unbundle By Name(w954) -> ("DataBase_array"=w953:T24)
            n403 = Not(x=w966) -> (.not. x?=w963:bool)
            n404 = Compound Arithmetic op=AND(w964, w963) -> (w962:bool)
            n405 = case shown="真" w962 {
              tunnel: ["Unload_LDF fail " ("消息") "Unload_LDF successful " ("消息")] -> w955
              frame False {
              }
              frame True {
                n406 = control-ref of="Tree control"() -> (w974:refnum<vi>)
                n407 = local write "Laod LDF Successful?"(FALSE ("Laod LDF Successful?")) -> ()
                n408 = invoke class="Tree (严格)" method="Edit Tree Items.Delete"(reference=w974) -> ()  [unwired: 4 in, 5 out]
              }
            }
            n409 = property class="Arr (严格)"(reference=w953, "Value"=T1 [] ("值")) -> ()  [unwired: 1 in, 2 out]
            n410 = One Button Dialog(message=w955) -> ()  [unwired: 1 in, 1 out]
            n411 = call "Log.vi"("Data"=w955) -> ()  [unwired: 3 in]
            n412 = To Variant(anything=w954) -> (Variant=w960:variant)
            n413 = Bundle By Name(cluster=T26 {"Sender"="", "receiver"="", "message"="", "data"=variant, "LIN Data array"=[]} ("Communication message"), "message"="Config update" ("Communication message.message"), "data"=w960) -> (w957:T26)
            n414 = Enqueue Element(queue=w959, element=w957, error in (no error)=w958) -> ()  [unwired: 1 in, 3 out]
          }
          frame "Start Log" {
            n415 = Unbundle By Name(w976) -> ("LIN_Data.DLL_PATH"=w985:path, "LIN_Data.Blf_Log.Blf_Log_PATH"=w977:path)
            n416 = Path To String(path=w977) -> (string=w978:string)
            n417 = call "tsapp_start_logging.vi"("AFullFileName"=w978, "路径输入"=w985) -> ("error out"=w983:errorcluster, "retuen"=w984:i32)  [unwired: 7 in, 1 out]
            n418 = Equal To 0?(x=w984) -> (x = 0?=w982:bool)
            n419 = Select(t=" Start Log Successful ", s=w982, f=" Start Log Fail ") -> (s? t:f=w979:string)
            n420 = Bundle By Name(cluster=w976, "error in"=w983) -> (w975:T18)
            n421 = call "Log.vi"("Data"=w979) -> ()  [unwired: 3 in]
          }
          frame "Stop Log" {
            n422 = Unbundle By Name(w989) -> ("LIN_Data.DLL_PATH"=w992:path)
            n423 = call "tsapp_stop_logging.vi"("Path"=w992) -> ("error out"=w990:errorcluster, "retuen"=w991:i32)  [unwired: 8 in, 1 out]
            n424 = Equal To 0?(x=w991) -> (x = 0?=w996:bool)
            n425 = Select(t=" Stop Log Successful ", s=w996, f=" Stop Log Fail ") -> (s? t:f=w993:string)
            n426 = Bundle By Name(cluster=w989, "error in"=w990) -> (w988:T18)
            n427 = call "Log.vi"("Data"=w993) -> ()  [unwired: 3 in]
          }
          frame "Quit" {
            n428 = Current VI's Path() -> (path=w1009:path)
            n429 = Strip Path(path=w1009) -> (stripped path=w1004:path)  [unwired: 1 out]
            n430 = Bundle By Name(cluster=T26 {"Sender"="", "receiver"="", "message"="", "data"=variant, "LIN Data array"=[]} ("Communication message"), "message"="Quit") -> (w1011:T26)
            n431 = Unbundle By Name(w1019) -> ("LIN_Data.DLL_PATH"=w1015:path, "LIN_Data"=w1018:T19, "Communication message.Sender"=w1008:string, "AsynCall?"=w999:bool)
            n432 = Build Path(base path=w1004, name or relative path="data") -> (appended path=w1003:path)
            n433 = Enqueue Element(queue=w1014, element=w1011, error in (no error)=w1013) -> (error out=w1001:errorcluster)  [unwired: 1 in, 2 out]
            n434 = flat-sequence {
              tunnel: w1001 -> [w1032]
              tunnel: [w1032] -> w1000
              frame #0 {
                n435 = Wait (ms)(milliseconds to wait=u32 50 ("等待时间（毫秒）")) -> ()  [unwired: 1 out]
              }
            }
            n436 = Generate User Event(user event=w1006, event data cluster="Quit" ("y")) -> ()  [unwired: 2 in, 2 out]
            n437 = call "TSLIN_Configuration_Save.vi"("path"=w1003, "error in (no error)"=w1000, "Config Name"=w1008, "Read/Write"=enum16{"Read", "Write"}."Write", "LIN_Data"=w1018) -> ("error in (no error) 2"=w1016:errorcluster)  [unwired: 4 in, 2 out]
            n438 = case shown="假" w999 {
              tunnel: w1016 -> [w1025 w1031]
              tunnel: w1015 -> [w1027 _]
              tunnel: [w1030 w1031] -> w1005
              frame False {
                n439 = call "tsdb_unload_lin_dbs.vi"("error in (no error)"=w1025, "路径输入"=w1027) -> ("error out"=w1024:errorcluster, "路径输出"=w1026:path)  [unwired: 7 in, 1 out]
                n440 = call "tsapp_disconnect.vi"("error in (no error)"=w1024, "Path"=w1026) -> ("error output"=w1028:errorcluster, "Path output"=w1029:path)  [unwired: 7 in, 1 out]
                n441 = call "finalize_lib_tsmaster.vi"("error in (no error)"=w1028, "Path"=w1029) -> ("error out"=w1030:errorcluster)  [unwired: 8 in, 1 out]
              }
              frame True {
              }
            }
            n442 = Bundle By Name(cluster=w1019, "error in"=w1005) -> (w1017:T18)
          }
        }
        n443 = Unbundle By Name(w171) -> ("message"=w174:string)
        n444 = Unbundle By Name(w167) -> ("error in"=w166:errorcluster)
        n445 = call "error_collect.vi"("error in (no error)"=w166) -> ("error IO"=w164:errorcluster)  [unwired: 10 in]
        n446 = case shown="\"default\", 默认" w174 {
          tunnel: w180 -> [w190 w192]
          tunnel: w179 -> [w186 w191]
          tunnel: [w189 w192] -> w177
          tunnel: [w188 w191] -> w176
          tunnel: w171 -> [w187 _]
          frame "default", Default {
            n447 = Enqueue Element(queue=w190, element=w187, error in (no error)=w186) -> (queue out=w189:refnum<queue>, error out=w188:errorcluster)  [unwired: 1 in, 1 out]
          }
          frame "" {
          }
        }
        n448 = Bundle By Name(cluster=w167, "error in"=w164) -> (w165:T18)
      }
    }
  }
  n449 = Release Queue(queue=w5, error in (no error)=w4) -> ()  [unwired: 1 in, 3 out]
  n450 = Destroy User Event(user event=w2) -> (error out=w3:errorcluster)  [unwired: 1 in]
  n451 = Release Queue(queue=w9, error in (no error)=w8) -> (error out=w10:errorcluster)  [unwired: 1 in, 2 out]
  n452 = property class="App"(error in=w10) -> (error out=w7:errorcluster, "App.Kind"=w6:T29)  [unwired: 1 in, 1 out]
  n453 = Unregister For Events(event registration refnum=w1, error in=w3) -> ()  [unwired: 1 out]
  n454 = case shown="\"Run Time System\"" w6 {
    tunnel: w7 -> [_ _ w1220 _ _ _ _]
    frame "invalid app kind", Default {
    }
    frame "Development System" {
    }
    frame "Run Time System" {
      n455 = invoke class="VI" method="FP.Close"(error in=w1220) -> ()  [unwired: 2 in, 3 out]
    }
    frame "Student Edition" {
    }
    frame "Embedded LabVIEW" {
    }
    frame "Evaluation" {
    }
    frame "Custom" {
    }
  }
